vi "Forebrain - Final.vi"() -> ()   [LabVIEW 2012]
doc: "This VI contrains the Forebrain within the Olin Robot Architecture. It must be run first to load the appropriate mission definition files. It contains a finite state machine built around a tabbed Operator interface that will guide an operator through the startup, run shutdown mission sequence. After running it, run the Midbrain and Hindbrain VIS."
panel:
  in  "MapDarWithBuoys?":bool
  out "under cloud?":bool
  out "WhatAroundMeMap? Filtered":cluster{"T":dbl, "Range":dbl, "Bearing":dbl}[](array[cluster])
  out "Forebrain to Midbrain":T1
  in  "Upper Midbrain Active":bool
  out "Ir distance":i16
  in  "Midbrain Behavior weights":i8[](array[numeric])=[0, 0, 0, 0, 0, 0]
  in  "SOFT E-STOP":bool
  in  "Upper Midbrain Tweaks":T2={"Lider good scale mult"=0.00125, "Lider good scale add"=0.0, "Lider speed scale mult"=0.018, "Lider speed scale add"=0.0, "Follow right?"=FALSE, "IR Following Distance"=400, "IR scaling div"=50.0, "Lidar Cutoff"=0.0}
  out "Normalized Buoy Array":i32[][](array[numeric])
  in  "Buoy Array":i32[][](array[numeric])
  out "Number Waypoints":i32
  out "NXT String Sent":string="$B^"
  in  "Soft E-Stop":bool
  out "NXT String Received":string
  out "return count":u32
  out "error out":errorcluster
  in  "error in 2":errorcluster
  out "Desired \nVelocity":i16=5
  out "Ycurrent":dbl format="%#_3g"
  out "Xcurrent":dbl format="%#_3g"
  out "Ystart":dbl
  out "Xstart":dbl
  in  "error in":errorcluster
  out "Robot Live":bool
  in  "E-Stop":bool
  in  "Tab":T3(tab)
  out "MissionTime (Min)":dbl(knob) scale=0.0..10.0
  out "LidarDist":i16
  out "IR Index":i32
  out "BatteryLevel":dbl(slide) scale=6.0..9.0
  out "String Received":string
  out "Send String":string="$B^"
  in  "VISA resource name":refnum<visa-resource-name>="COM6"
  in  "Mode":i16 min=0 max=99 step=1
  in  "Desired Vel":i16(slide)=7 scale=0.0..14.0
  in  "Local Head":i16(slide)=7 scale=0.0..14.0
  out "StartMissionMap":picture
  out "MapDARCheck":picture
  in  "RunRobot":bool
  in  "Tug letter":string="G"
  out "Tug X":i32
  out "Tug Y":i32
  out "Tug H":i32
  out "BS Time Out?":bool
  out "Buoy locations":cluster{"regular expression":string, i32, i32}[](array[cluster])
  out "Valid ?":bool
  out "Battery\nVolts":i16
  out "Base Station data rec'd":string
  out "udp rate":bool
  out "CollisionWarning":bool
  out "DebugMapDAR":picture
  in  "MapDAR Control":T4={"NumberOfBeams"=180, "SensorRange"=500.0, "Noise (0.1 to 1)"=0.0} {"Noise (0.1 to 1)" min=0.0 max=1.0 step=0.1; "SensorRange" min=500.0 max=1500.0 step=100.0; "NumberOfBeams" min=36 max=360 step=2}
  out "MapDAR Data (r:pixel b:degrees)":cluster{"Range":dbl, "Bearing":dbl}[](array[cluster])
  in  "Stop DebugSENSE":bool
  out "MissionMap":picture
  out "Tug position":T5
  out "initialized MDF":T6(array[cluster])
  out "Way Point Index":i32
  out "InitialWaypoint":cluster{"X":i16, "Y":i16}
  in  "Pen Color":u32(colorbox)=15671808
  in  "Select Pen Attributes":T7={"Width"=1, "Style"=enum."Solid"}
  out "Draw??":bool
  in  "WhereAmI?FromBase":T8
  out "(xr,yr)":cluster{"X":dbl, "Y":dbl}
  in  "RobotPosition":T5 {"xrobot" min=0.0 max=1177.0 step=10.0; "yrobot" min=0.0 max=850.0 step=10.0; "heading" min=0.0 max=7.0 step=0.1}
  out "MDF_Original":T6(array[cluster])
  out "WhatAroundMeMap?":cluster{"T":dbl, "Range":dbl, "Bearing":dbl}[](array[cluster])
  out "WayPointAct":dbl[](array[numeric])
  out "SteerAngle":dbl
  out "MissionDefFile":picture
  out "MDF":T6(array[cluster])
  in  "Select Your Behavior":T9(ring)
  out "No. of Waypoints":i32
  in  "Exit Planning":bool
  in  "BoatSpeed for Leg":dbl(slide)=8.0 min=-9.0 max=9.0 step=1.0 scale=0.0..14.0
  out "BuildMDF":bool
  out "WayPoint Position":cluster{"X":i32, "Y":i32}
  out "Send String to NXT":string="$B^"
  in  "Behavior Command":T9(ring)
  out "CollisionLight":bool
  out "Where? Manual":T8
  out "ActManual":bool
  in  "Manual Heading":i16(knob)=7 min=0 max=14 step=1
  out "MWhat?":bool
  out "Where? 2":bool
  out "How? 2":bool
  in  "ManualModeStop":bool
  out "ManualModeMapDAR":picture
  out "ManualMissionMap":picture
  out "Battery":dbl(slide) scale=0.0..8.0
  in  "Manual Vel":dbl(slide)=7.0 min=0.0 max=14.0 step=1.0 scale=0.0..14.0
  out "MissionTime":dbl(knob) scale=0.0..10.0
  out "Heading":cluster{dbl, dbl}(knob)={0.0, 34.390870865624734} scale=180.0..-179.0 scale format="%#_3g"
  out "Speed":i16(knob) scale=-6.0..6.0
  out "Current Behavior":T9(ring)
  out "Robot Position":cluster{"X":dbl, "Y":dbl} {"X" format="%#_3g"; "Y" format="%#_3g"}
  out "Ready":bool
  in  "Pause":bool
  in  "Rerun MDF":bool
  out "CollisionLight 2":bool
  out "Act":bool
  out "Neo-C":bool
  out "How?":bool
  out "What?":bool
  out "A Heading":cluster{dbl, dbl}(knob)={0.0, 34.390870865624734} scale=180.0..-180.0
  out "A Speed":dbl(knob) scale=-9.0..9.0
  out "AutoBattery":dbl(slide) scale=0.0..8.0
  out "AutoModeLIDAR":picture
  out "AutoMissionMap":picture
  in  "RunAutoMode":bool
  out "MissionTimeAuto":dbl(knob) scale=0.0..60.0
  out "Where?":bool
  in  "WAYPOINT\n MODE":dbl=1.0
  in  "Current Waypoint":dbl
  in  "Manual\nOverride":bool=TRUE
  in  "Destinations Array":i64[][](array[numeric])=[[120, 280, 700, 408], [30, 140, 250, 400], [217, 811, 641, 816]]
  out "BAM Mission Map":picture
  out "Pixel X":dbl
  out "Pixel Y":dbl
  out "Direction":dbl
  out "Base Station String":string
  out "Battery Level":dbl
  in  "Heading":i16(knob)=7
  in  "Velocity":i16(slide)=7 scale=0.0..14.0
  out "Local\nHeading":i16=90
  # "To run\nrobot,\nclick\narrow\nabove\n\nRun Robot button must be on"
  # "Operation Directions\n\n1)Click on Startup&\nShutdown tab.\n2) Click on Run \nArrow on menubar.\nRun Forebrain,\nvis from the project\nexplorer.\n3) Select a mssion \nmap file when asked.\n4) Check robot is \nfully operational on\nStartup tab.\n5) Debug with debug\ntabs as required.\n6) Select ManualMode\ntab and test drive \nrobot.\n7) Select PlanMission\ntab and set up \nmission.\n8) Go to AutoMode\ntab and run mission."
  # "Turns off drive\nmotors"
  # "forebrain"
  # "wall follow"
  # "wall avoid"
  # "under cloud"
  # "GTFO"
  # "tend straight"
  # "inactive behaviors = 0\nstrongest behavior = 10"
  # "under cloud should always be zero"
  # "under cloud?"
  # "Enter Olin Test  Pool"
  # "Xbee Com Port"
  # "xBee\"Send String\" (mode, desired velocity, local heading)"
  # "(Type in Tug Letter  L T G P  (look at boat cradle)"
  # "Should be on to\nrun"
  # "BoatG,X,Y,H,BoatT,X,Y,H,BoatP,X,Y.H,BoatL,X,Y,H,BuoyA,X,Y,BuoyB,X,Y,BuoyC,X,Y,BuoyD,X,Y,Time(hours,Min,Sec)"
  # "To stop  program \nturn off here"
  # "Use this tab\nto explore\nLIDAR\ndata and \noperation"
  # "Set\nNumberOfBeams\nSensorRange\nNoise\nto\nview\nsimulated\nsensor\ndata"
  # "Turn Debug Sim \nto leave this\ntab--->"
  # "This tab will auto\nreturn to Startup \nin 2 seconds"
  # "Clean up interface and make more useful for debugging behaviors"
  # "Build out interface and make more useful for debugging act"
  # "This tab will auto\nreturn to Startup \nin 2 seconds"
  # "Directions:\n1) Select Robot Behavior for each mission leg.\n2) Select Robot Speed for leg.\n3) Click on robots current location for first waypoint.\n4) Hold down button and drag to next\nwaypoint. Click on next leg waypoint.\n5) Hold mouse button down and drag to \nnext waypoint. \n6) Click on next waypoint. Repeat for full mission.\n7) MDF will store up to 20 waypoints."
  # "Remember to\nset boat\nleg speed !"
  # "Please Adjust Scroll Barrs in Tug Off Mode to Prevent  Extra Lines Being Drawn"
  # "\"Send String\" (mode, desired velocity, local heading)"
  # "Press to stop and return to StartUp"
  # "Open MidBrain\nArbiter to see\nBrain Waves"
  # "AutoMode\nAutomatically \nReturns to \nStartUp Mode"
  # "Pixel coordinates for destinations."
  # "BoatG,X,Y,H,BoatT,X,Y,H,BoatP,X,Y.H,BoatL,X,Y,H,BuoyA,X,Y,BuoyB,X,Y,BuoyC,X,Y,BuoyD,X,Y,Time(hours,Min,Sec)"
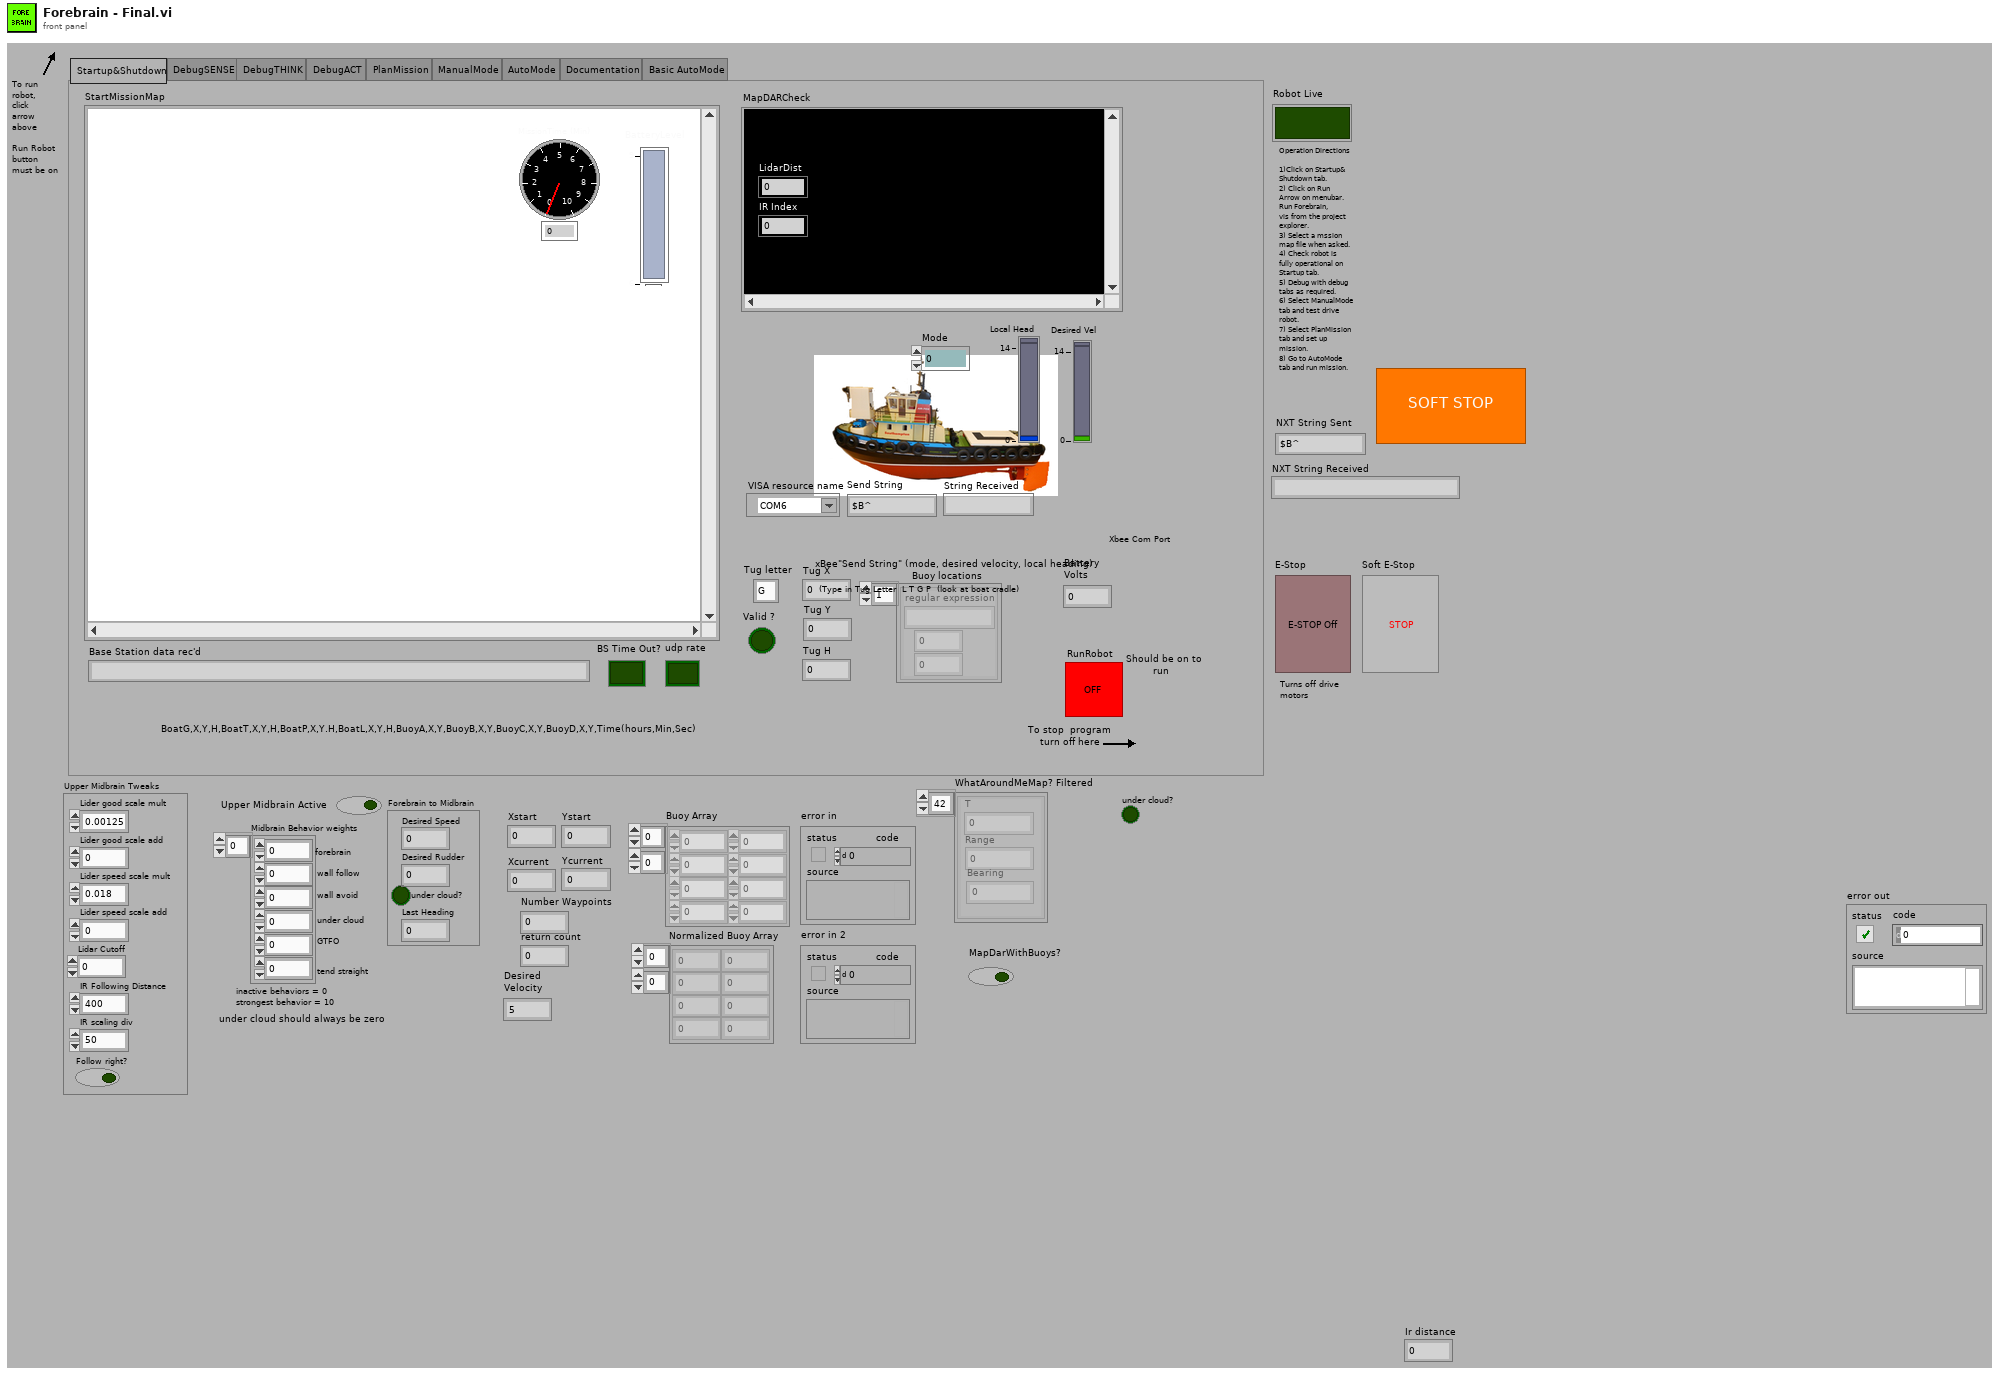
[diagram p1: front panel]
types:
  T1 = cluster{"Desired Speed":i16, "Desired Rudder":i16, bool, "Last Heading":i16}
  T2 = cluster{"Lider good scale mult":dbl, "Lider good scale add":dbl, "Lider speed scale mult":dbl, "Lider speed scale add":dbl, "Follow right?":bool, "IR Following Distance":i32, "IR scaling div":dbl, "Lidar Cutoff":dbl}
  T3 = enum32{"Startup&Shutdown", "DebugSENSE", "DebugTHINK", "DebugACT", "PlanMission", "ManualMode", "AutoMode", "Documentation", "Basic AutoMode"}
  T4 = cluster{"NumberOfBeams":i32, "SensorRange":dbl, "Noise (0.1 to 1)":dbl}
  T5 = cluster{"xrobot":dbl, "yrobot":dbl, "heading":dbl}
  T6 = cluster{"Status":enum16{"Past", "Current", "Future"}, "x":dbl, "y":dbl, "z":dbl, "Vel":dbl, "Dwell Time":dbl, "BehCom":enum16{"Tug Off", "Manual Mode", "Goto WayPoint", "Back Up", "Circle", "Left Wall Follow", "Right Wall Follow", "Hunt"}, "Expand1":dbl, "Expand2":dbl, "Expand3":dbl}[]
  T7 = cluster{"Width":u16, "Style":enum32{"Solid", "Dash", "Dot", "DashDot", "DashDotDot"}}
  T8 = cluster{"T":dbl, "X":dbl, "Y":dbl, "Direction":dbl}
  T9 = enum16{"Tug Off", "Manual Mode", "Goto WayPoint", "Back Up", "Circle", "Left Wall Follow", "Right Wall Follow", "Hunt"}
  T10 = enum32{"Startup&Shutdown", "DebugSENSE", "DebugTHINK", "DebugACT", "PlanMission", "ManualMode", "AutoMode", "Documentation"}
  T11 = cluster{"VelCom":dbl, "BehCom":enum16{"OpenFieldTransit", "P-WallFollow", "S-WallFollow", "LaneFollow", "ManualMode"}}
  T12 = typedef "IMAQ Image.ctl" = refnum<image>
  T13 = typedef "imagedata.ctl" = cluster{"image type":i32, "image depth":i32, "image":u8[], "mask":u8[], "colors":u32[], "Rectangle":cluster{"left":i16, "top":i16, "right":i16, "bottom":i16}}
  T14 = cluster{"Status":enum16{"Past", "Current", "Future"}, "x":dbl, "y":dbl, "z":dbl, "Vel":dbl, "Dwell Time":dbl, "BehCom":enum16{"Tug Off", "Manual Mode", "Goto WayPoint", "Back Up", "Circle", "Left Wall Follow", "Right Wall Follow", "Hunt"}, "Expand1":dbl, "Expand2":dbl, "Expand3":dbl}
  T15 = typedef "LVMouseTypeDef.ctl" = cluster{"Mouse Position":cluster{"X":i32, "Y":i32}, "Mouse Modifiers":cluster{"Button Down":bool, "Shift Mod":bool, "Menu Mod":bool, "Option Mod":bool}}
  T16 = cluster{"RudderAngle":i16, "t":i16, "under cloud?":bool, "Heading":i16}
  T17 = cluster{"regular expression":string, i32, i32, i32}
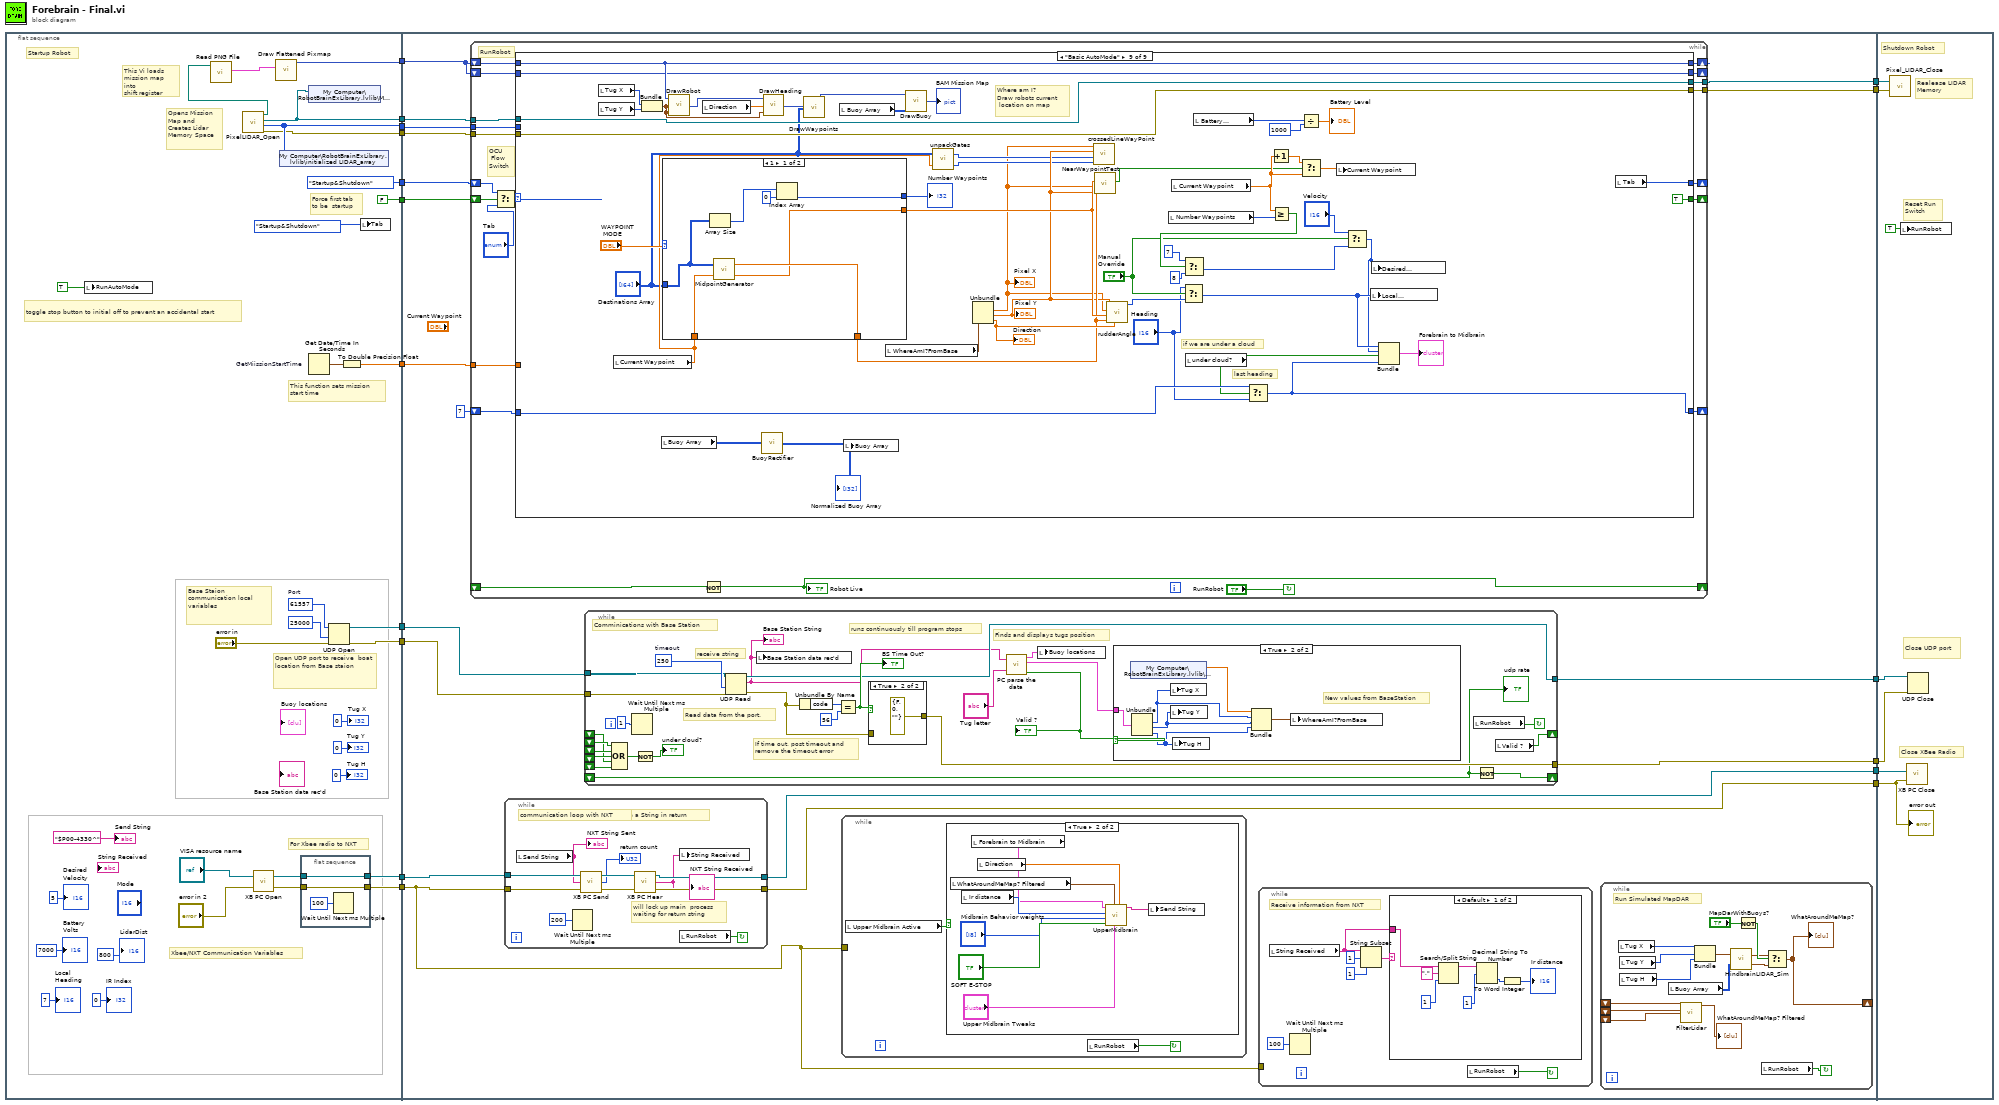
[diagram p0: block diagram]
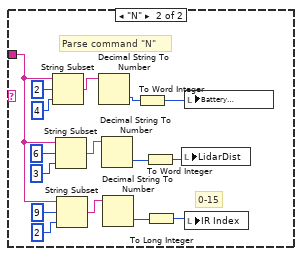
[diagram p2: hidden frame]
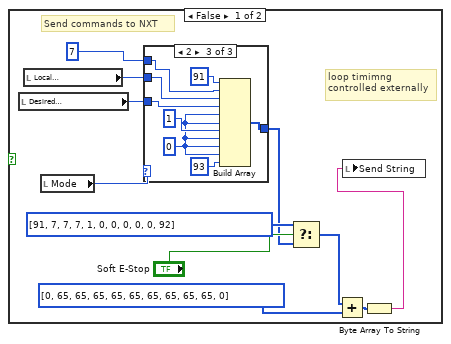
[diagram p3: hidden frame]
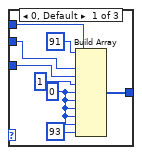
[diagram p4: hidden frame]
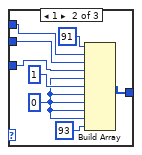
[diagram p5: hidden frame]
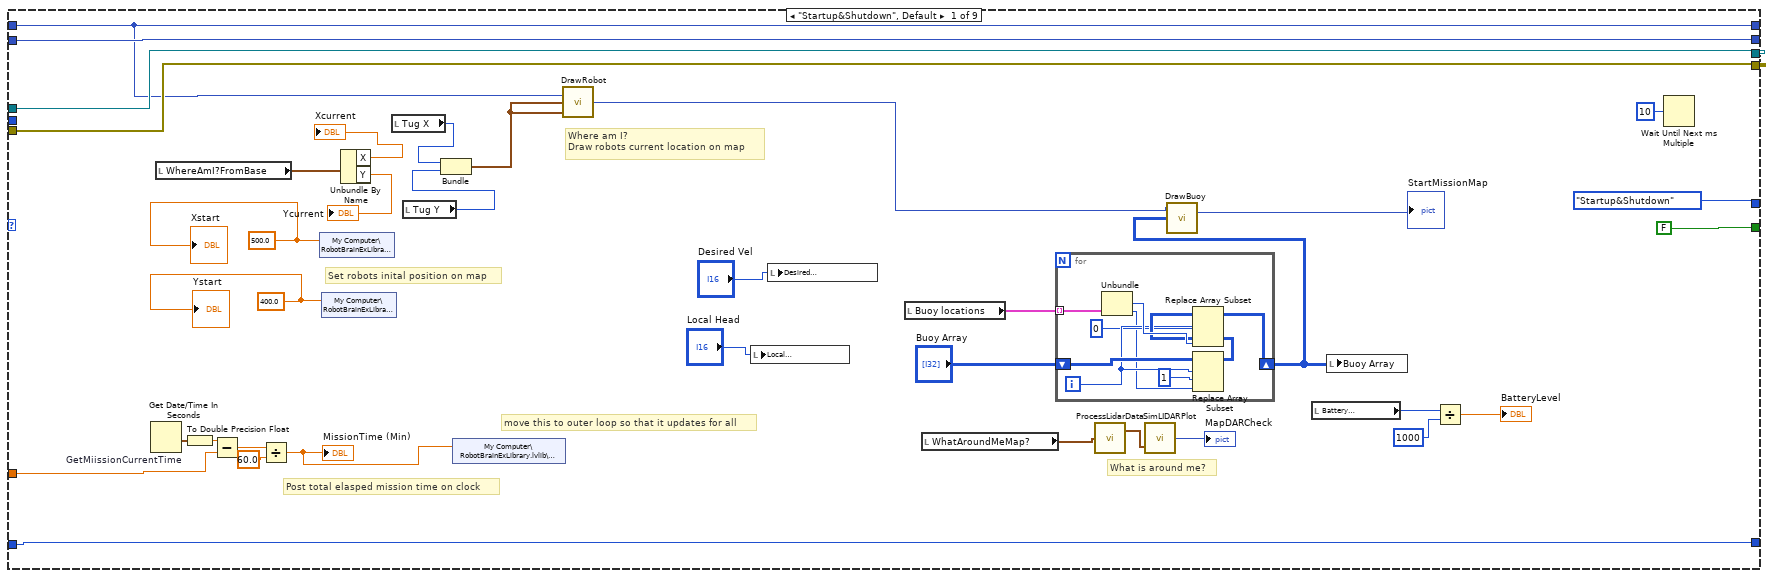
[diagram p8: hidden frame]
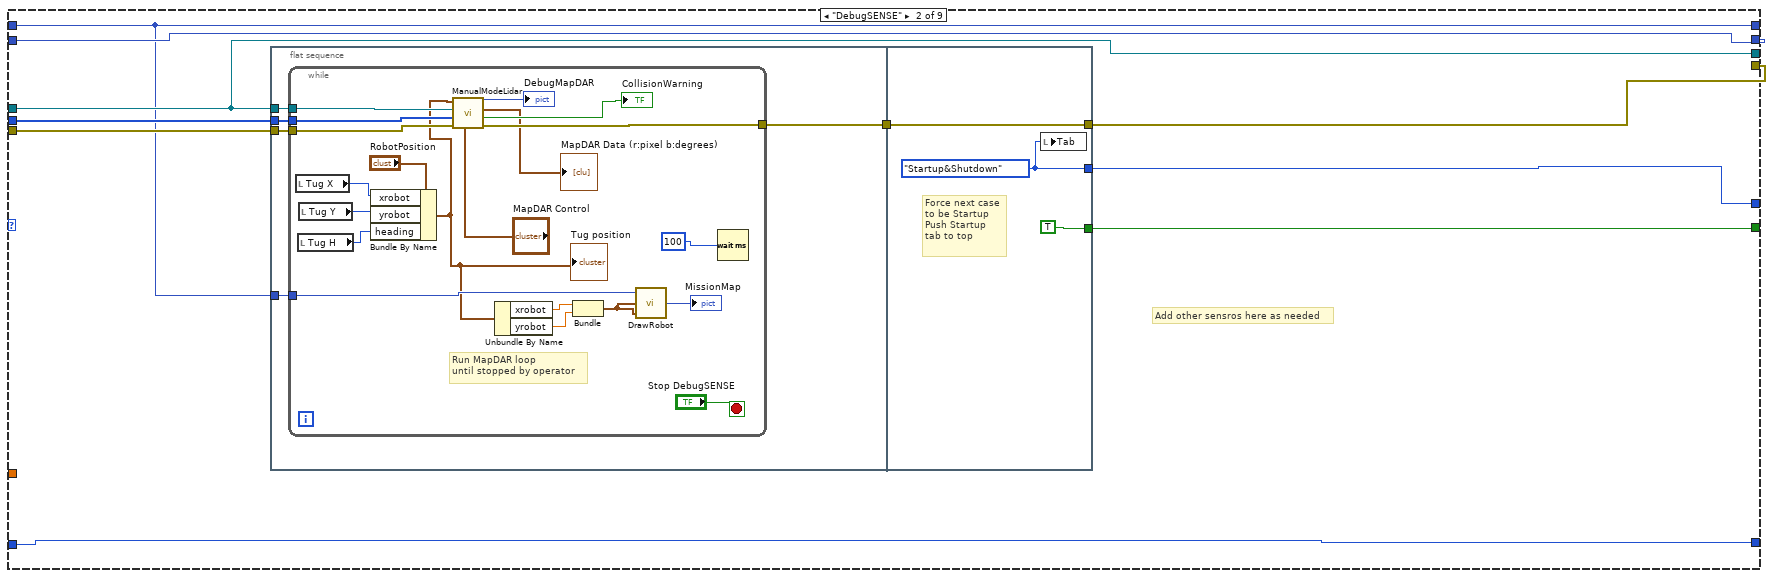
[diagram p9: hidden frame]
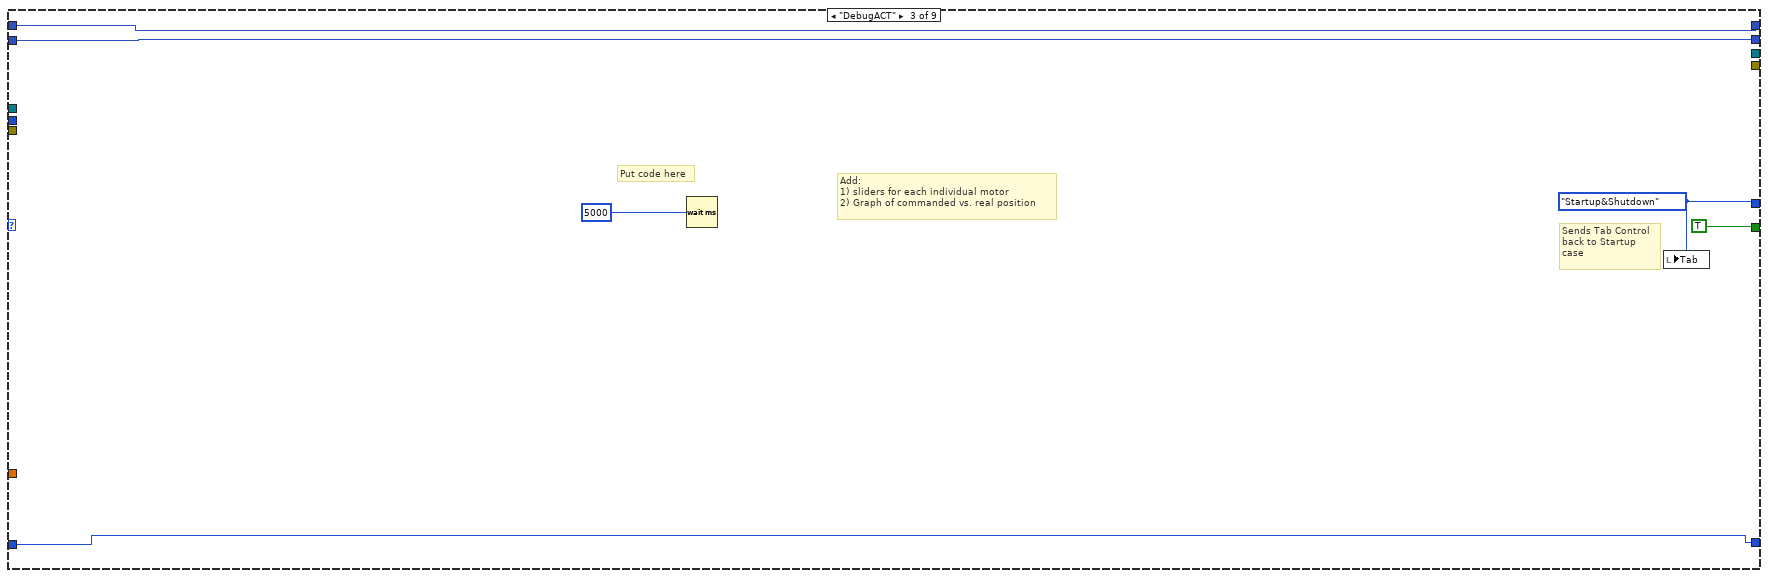
[diagram p10: hidden frame]
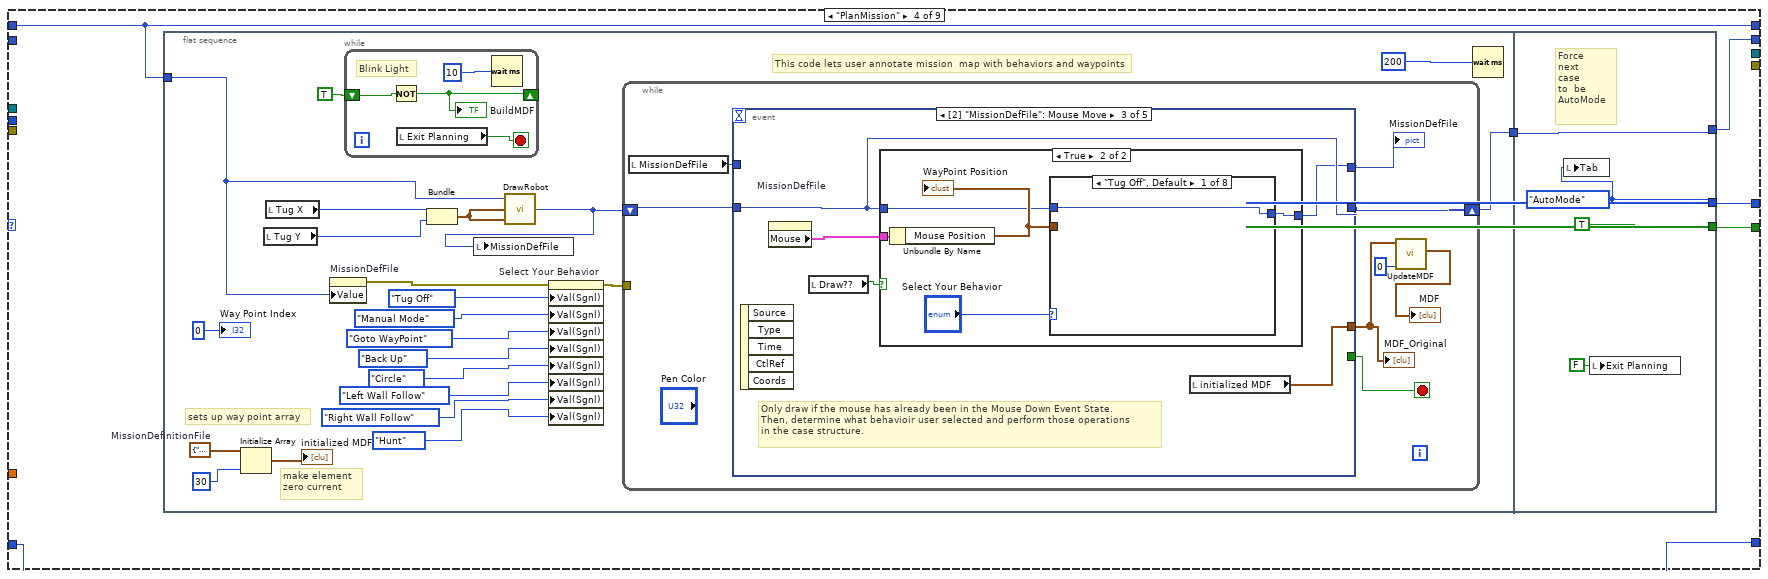
[diagram p11: hidden frame]
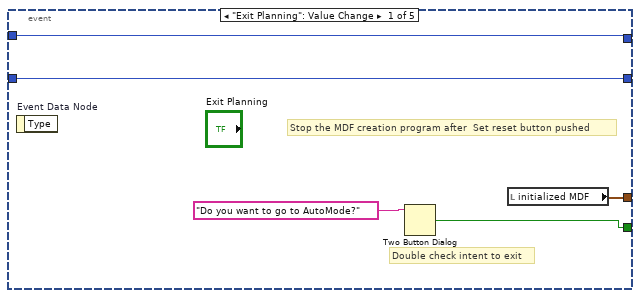
[diagram p12: hidden frame]
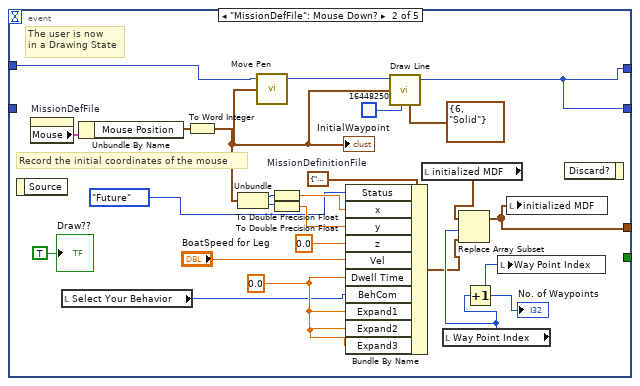
[diagram p13: hidden frame]
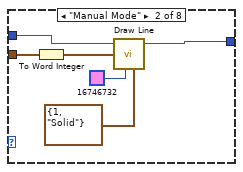
[diagram p15: hidden frame]
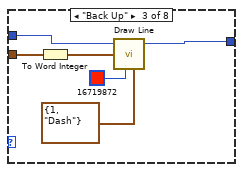
[diagram p16: hidden frame]
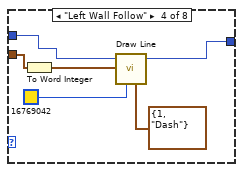
[diagram p17: hidden frame]
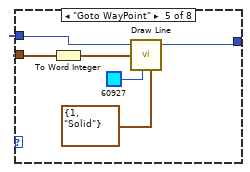
[diagram p18: hidden frame]
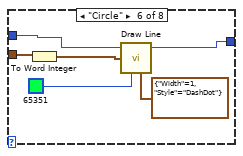
[diagram p19: hidden frame]
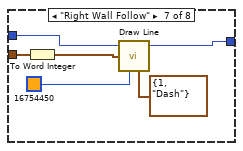
[diagram p20: hidden frame]
diagram:
  n1 = flat-sequence {
    tunnel: [w48] -> w17
    tunnel: [w47] -> w16
    tunnel: [w44] -> w15
    tunnel: [w46] -> w14
    tunnel: [w45] -> w13
    tunnel: [FALSE ("RunAutoMode")] -> w10
    tunnel: [T10."Startup&Shutdown" ("Tab")] -> w9
    tunnel: [w31] -> w8
    tunnel: [w30] -> w7
    tunnel: [w19] -> w6
    tunnel: [w18] -> w5
    tunnel: w17 -> [w70]
    tunnel: w16 -> [w69]
    tunnel: w15 -> [w68]
    tunnel: w14 -> [w67]
    tunnel: w13 -> [w66]
    tunnel: [w65] -> w12
    tunnel: [w64] -> w11
    tunnel: w10 -> [w63]
    tunnel: w9 -> [w62]
    tunnel: w8 -> [w57]
    tunnel: w7 -> [w56]
    tunnel: w6 -> [w61]
    tunnel: w5 -> [w58]
    tunnel: [w60] -> w4
    tunnel: [w59] -> w3
    tunnel: [w55] -> w2
    tunnel: [w54] -> w1
    tunnel: w12 -> [w738]
    tunnel: w11 -> [w737]
    tunnel: w4 -> [w736]
    tunnel: w3 -> [w735]
    tunnel: w2 -> [w734]
    tunnel: w1 -> [w733]
    frame #0 {
      w37 = u16 61557  # Port
      # "For Xbee radio to NXT"
      # "Xbee/NXT Communication Variables"
      # "Base Staion communication local variables"
      # "Open UDP port to receive  boat location from Base staion"
      # "Force first tab\nto be  startup"
      # "toggle stop button to initial off to prevent an accidental start"
      # "Opens Mission\nMap and\nCreates Lidar\nMemory Space"
      # "This function sets mission \nstart time"
      # "This Vi loads\nmission map into \nshift register"
      # "Startup Robot"
      n2 = local write "RunAutoMode"(TRUE ("RunAutoMode")) -> ()
      n3 = call "PixelLIDAR_Open.vi"() -> ("error out"=w45:errorcluster, "initialized LIDAR\narray"=w46:i32[], "MDF Image"=w44:T12, "MissionMap"=w39:path)  [unwired: 2 in]
      n4 = call <vilib>:"Read PNG File.vi"("path to PNG file"=w39) -> ("image data"=w38:T13)  [unwired: 8 in, 2 out]
      n5 = call "XB PC Open.vi"("error in (no error)"="error in 2", "VISA resource name"="VISA resource name") -> ("error out"=w22:errorcluster, "VISA resource name out"=w23:refnum<visa-resource-name>)
      n6 = call <vilib>:"Draw Flattened Pixmap.vi"("image data"=w38) -> ("new picture"=w47:picture)  [unwired: 8 in]
      n7 = shared-variable "My Computer\\RobotBrainExLibrary.lvlib\\initialized LIDAR_array"(w46) -> ()  [unwired: 1 in, 1 out]
      n8 = flat-sequence {
        tunnel: w23 -> [w50]
        tunnel: w22 -> [w51]
        tunnel: [w51] -> w18
        tunnel: [w50] -> w19
        frame #0 {
          n9 = Wait Until Next ms Multiple(millisecond multiple=u32 100) -> ()  [unwired: 1 out]
        }
      }
      n10 = shared-variable "My Computer\\RobotBrainExLibrary.lvlib\\MDF Image"(w44) -> ()  [unwired: 1 in, 1 out]
      n11 = Get Date/Time In Seconds "GetMiissionStartTime"() -> (seconds since 1Jan1904=w49:timestamp)
      n12 = UDP Open(8:"error in", 9:25000 ("timeout ms (25000)"), 11:w37) -> (port=w31:refnum<k16>, 0:w30:errorcluster)  [unwired: 2 in, 1 out]
      n13 = To Double Precision Float(number=w49) -> (double precision float=w48:dbl)
      n14 = local write "Tab"(T10."Startup&Shutdown" ("Tab")) -> ()
      "Tug X" <- 0 ("Tug X")
      "Tug Y" <- 0 ("Tug Y")
      "Tug H" <- 0 ("Tug H")
      "Battery\nVolts" <- i16 7000 ("Battery\nVolts")
      "LidarDist" <- i16 800 ("Dist")
      "IR Index" <- 0 ("IR Index")
      "Local\nHeading" <- i16 7 ("Local\nHeading")
      "Desired \nVelocity" <- i16 5 ("Desired \nVelocity")
      "Send String" <- "$P00-4330^"
    }
    frame #1 {
      n15 = while {
        shift-right: [w208] -> _
        shift-left: _ -> [w224]
        shift-right: [w223] -> _
        shift-left: w62 -> [w222]
        shift-right: [w219] -> _
        shift-left: w63 -> [w218]
        tunnel: w70 -> [w217]
        shift-right: [w207] -> _
        shift-left: w69 -> [w216]
        shift-right: [w214] -> _
        shift-left: w69 -> [w215]
        tunnel: w68 -> [w213]
        tunnel: w67 -> [w212]
        tunnel: w66 -> [w211]
        tunnel: [w210] -> w65
        tunnel: [w209] -> w64
        shift-right: [w206] -> _
        shift-left: i16 7 ("Heading") -> [w205]
        stop <- "RunRobot" continue-if-true
        # "RunRobot"
        # "OCU\n Flow\nSwitch"
        n16 = Select(t=w222, s=w218, f="Tab") -> (s? t:f=w220:T3)
        n17 = case shown="\"Basic AutoMode\"" w220 {
          selector: w220 -> [_ _ _ _ _ w563 _ _ _]
          tunnel: [T10."Startup&Shutdown" ("Tab") w275 w311 w319 w487 w564 T10."Startup&Shutdown" ("Tab") w662 w704] -> w223
          tunnel: [FALSE ("s") w274 TRUE ("s") w318 w488 w562 FALSE ("s") TRUE ("s") TRUE ("s")] -> w219
          tunnel: w217 -> [w254 _ _ _ w485 w560 _ _ _]
          tunnel: w216 -> [w232 w271 w310 w315 w483 w557 w654 w660 w710]
          tunnel: w215 -> [w253 w272 w309 _ w484 w559 w653 w659 w709]
          tunnel: [w253 w272 w309 w316 w484 w559 w653 w659 w709] -> w214
          tunnel: w213 -> [w252 w273 _ _ _ _ _ _ w705]
          tunnel: w212 -> [_ w279 _ _ _ _ _ _ _]
          tunnel: w211 -> [w251 w278 _ _ _ _ _ _ w702]
          tunnel: [w252 w273 _ _ _ _ _ _ w705] -> w210
          tunnel: [w251 w277 _ _ _ _ _ _ w702] -> w209
          tunnel: [w232 w271 w310 w315 w483 w557 w654 w660 w710] -> w207
          tunnel: [w226 w270 w308 w314 w482 w556 w652 w658 w672] -> w206
          tunnel: w205 -> [w226 w270 w308 w314 w482 w556 w652 w658 w674]
          frame "Startup&Shutdown", Default {
            w243 = 400.0 ("Ystart")
            w244 = 500.0 ("Xstart")
            # "move this to outer loop so that it updates for all"
            # "Where am I?\nDraw robots current location on map"
            # "Post total elasped mission time on clock"
            # "What is around me?"
            # "Set robots inital position on map"
            n18 = Get Date/Time In Seconds "GetMiissionCurrentTime"() -> (seconds since 1Jan1904=w258:timestamp)
            n19 = local read "WhereAmI?FromBase"() -> (w233:T8)
            n20 = To Double Precision Float(number=w258) -> (double precision float=w257:dbl)
            n21 = Subtract(x=w257, y=w254) -> (x-y=w256:dbl)
            n22 = Divide(x=w256, y=60.0) -> (x/y=w250:dbl)
            "MissionTime (Min)" <- w250
            n23 = shared-variable "My Computer\\RobotBrainExLibrary.lvlib\\Xstart"(w244) -> ()  [unwired: 1 in, 1 out]
            n24 = shared-variable "My Computer\\RobotBrainExLibrary.lvlib\\Ystart"(w243) -> ()  [unwired: 1 in, 1 out]
            n25 = Unbundle By Name(w233) -> ("X"=→"Xcurrent":dbl, "Y"=→"Ycurrent":dbl)
            n26 = local read "Tug X"() -> (w242:i32)
            n27 = local read "Tug Y"() -> (w241:i32)
            n28 = Bundle("Tug X"=w242, "Tug Y"=w241) -> (w247:cluster{"Tug X":i32, "Tug Y":i32})  [unwired: 1 in]
            n29 = shared-variable "My Computer\\RobotBrainExLibrary.lvlib\\MissionTime"(w250) -> ()  [unwired: 1 in, 1 out]
            n30 = call "DrawRobot.vi"("(xr,yr) old"=w247, "(xr,yr) new"=w247, "2D Picture"=w232) -> ("new picture"=w231:picture)
            n31 = local write "Local\nHeading"("Local Head") -> ()
            n32 = local write "Desired \nVelocity"("Desired Vel") -> ()
            n33 = local read "Buoy locations"() -> (w229:cluster{"regular expression":string, i32, i32}[])
            n34 = local read "WhatAroundMeMap?"() -> (w234:cluster{"T":dbl, "Range":dbl, "Bearing":dbl}[])
            n35 = for {
              tunnel: w229 -> [w269] mode=indexing
              shift-right: [w265] -> w227
              shift-left: "Buoy Array" -> [w268]
              i -> [w263]
              n36 = Unbundle(w269) -> (w267:i32, w261:i32)  [unwired: 1 out]
              n37 = Replace Array Subset(array=w268, new element=w261, index (row)=w263, index (col)=1 ("index")) -> (w266:i32[][])
              n38 = Replace Array Subset(array=w266, new element=w267, index (row)=w263, index (col)=0 ("index")) -> (w265:i32[][])
            }
            n39 = call "ProcessLidarData.vi"("WhatAroundMe?MM"=w234) -> ("data array [mag, phase (deg)]"=w248:cluster{"magnitude":dbl, "phase":dbl}[])  [unwired: 1 out]
            n40 = call "SimLIDARPlot.vi"("data array [mag, phase (deg)]"=w248) -> ("SONAR"=→"MapDARCheck":picture)  [unwired: 1 in]
            n41 = call "DrawBuoy.vi"("Array"=w227, "2D Picture"=w231) -> ("new picture"=→"StartMissionMap":picture)  [unwired: 1 in]
            n42 = local read "Battery\nVolts"() -> (w238:i16)
            n43 = local write "Buoy Array"(w227) -> ()
            n44 = Divide(x=w238, y=i16 1000) -> (x/y=→"BatteryLevel":dbl)
            n45 = Wait Until Next ms Multiple(millisecond multiple=u32 10) -> ()  [unwired: 1 out]
            "Xstart" <- w244
            "Ystart" <- w243
          }
          frame "DebugSENSE" {
            # "Add other sensros here as needed"
            n46 = flat-sequence {
              tunnel: w279 -> [w284]
              tunnel: w278 -> [w283]
              tunnel: w273 -> [w282]
              tunnel: [w281] -> w276
              tunnel: w271 -> [w280]
              tunnel: [w307] -> w277
              tunnel: w276 -> [w307]
              tunnel: [w306] -> w275
              tunnel: [TRUE ("s")] -> w274
              frame #0 {
                n47 = while {
                  tunnel: w284 -> [w304]
                  tunnel: w283 -> [w303]
                  tunnel: w282 -> [w302]
                  tunnel: [w301] -> w281
                  tunnel: w280 -> [w295]
                  stop <- "Stop DebugSENSE" stop-if-true
                  # "Run MapDAR loop\nuntil stopped by operator"
                  n48 = local read "Tug X"() -> (w289:i32)
                  n49 = local read "Tug H"() -> (w290:i32)
                  n50 = local read "Tug Y"() -> (w288:i32)
                  n51 = Bundle By Name(cluster="RobotPosition", "xrobot"=w289, "yrobot"=w288, "heading"=w290) -> (w286:T5)
                  "Tug position" <- w286
                  n52 = call "ManualModeLidar.vi"("LIDARControl"="MapDAR Control", "error in"=w303, "initialized \nsonar ray\narray"=w304, "MDF Image"=w302, "SubPosition"=w286) -> ("error out"=w301:errorcluster, "Collision\nWarning"=→"CollisionWarning":bool, "LIDAR Data (r:pixel b:degrees)"=→"MapDAR Data (r:pixel b:degrees)":cluster{"Range":dbl, "Bearing":dbl}[], "LIDAR"=→"DebugMapDAR":picture)  [unwired: 1 in]
                  n53 = Unbundle By Name(w286) -> ("xrobot"=w293:dbl, "yrobot"=w292:dbl)
                  n54 = Bundle("xrobot"=w293, "yrobot"=w292) -> (w285:cluster{"xrobot":dbl, "yrobot":dbl})  [unwired: 1 in]
                  n55 = call "DrawRobot.vi"("(xr,yr) old"=w285, "(xr,yr) new"=w285, "2D Picture"=w295) -> ("new picture"=→"MissionMap":picture)
                  n56 = Wait (ms)(milliseconds to wait=u32 100) -> ()  [unwired: 1 out]
                }
              }
              frame #1 {
                w306 = T10."Startup&Shutdown" ("Tab")
                # "Force next case\nto be Startup\nPush Startup\ntab to top"
                n57 = local write "Tab"(w306) -> ()
              }
            }
          }
          frame "DebugACT" {
            w311 = T10."Startup&Shutdown" ("Tab")
            # "Add:\n1) sliders for each individual motor\n2) Graph of commanded vs. real position"
            # "Put code here"
            # "Sends Tab Control\nback to Startup\ncase"
            n58 = Wait (ms)(milliseconds to wait=u32 5000) -> ()  [unwired: 1 out]
            n59 = local write "Tab"(w311) -> ()
          }
          frame "PlanMission" {
            n60 = flat-sequence {
              tunnel: [w340] -> w317
              tunnel: w315 -> [w333]
              tunnel: [w480] -> w319
              tunnel: [TRUE ("s")] -> w318
              tunnel: w317 -> [w479]
              tunnel: [w479] -> w316
              frame #0 {
                w331 = T14 {"Status"=enum."Future", "x"=0.0, "y"=0.0, "z"=0.0, "Vel"=0.0, "Dwell Time"=0.0, "BehCom"=enum."Tug Off", "Expand1"=0.0, "Expand2"=0.0, "Expand3"=0.0}  # MissionDefinitionFile
                # "make element \nzero current"
                # "sets up way point array"
                # "This code lets user annotate mission  map with behaviors and waypoints"
                n61 = Initialize Array ("Initialize WaypointArray")(w331, 30 ("dimension size")) -> (→"initialized MDF":T6)
                n62 = local read "Tug Y"() -> (w328:i32)
                n63 = local read "Tug X"() -> (w329:i32)
                n64 = property on="MissionDefFile" class="Pict"("Value"=w333) -> (error out=w338:errorcluster)  [unwired: 2 in, 1 out]
                n65 = while {
                  shift-right: [w344] -> _
                  shift-left: TRUE -> [w345]
                  stop <- w343 stop-if-true
                  # "Blink Light"
                  n66 = Not(x=w345) -> (.not. x?=w344:bool)
                  "BuildMDF" <- w344
                  n67 = local read "Exit Planning"() -> (w343:bool)
                  n68 = Wait (ms)(milliseconds to wait=u32 10) -> ()  [unwired: 1 out]
                }
                n69 = Bundle("Tug X"=w329, "Tug Y"=w328) -> (w334:cluster{"Tug X":i32, "Tug Y":i32})  [unwired: 1 in]
                n70 = call "DrawRobot.vi"("(xr,yr) old"=w334, "(xr,yr) new"=w334, "2D Picture"=w333) -> ("new picture"=w332:picture)
                n71 = local write "MissionDefFile"(w332) -> ()
                n72 = property on="Select Your Behavior" class="Enum (strict)"(error in=w338, "Val(Sgnl)"=T9."Tug Off" ("Value (Signaling)"), "Val(Sgnl)"=T9."Manual Mode" ("Value (Signaling)"), "Val(Sgnl)"=T9."Goto WayPoint" ("Value (Signaling)"), "Val(Sgnl)"=T9."Back Up" ("Value (Signaling)"), "Val(Sgnl)"=T9."Circle" ("Value (Signaling)"), "Val(Sgnl)"=T9."Left Wall Follow" ("Value (Signaling)"), "Val(Sgnl)"=T9."Right Wall Follow" ("Value (Signaling)"), "Val(Sgnl)"=T9."Hunt" ("Value (Signaling)")) -> (error out=w339:errorcluster)  [unwired: 1 in, 1 out]
                n73 = while {
                  shift-right: [w352] -> w340
                  shift-left: w332 -> [w353]
                  tunnel: w339 -> [_]
                  stop <- w351 stop-if-true
                  n74 = local read "MissionDefFile"() -> (w350:picture)
                  n75 = event shown="[2] \"MissionDefFile\": Mouse Move" {
                    selector: _ -> [_ _ _ _ _]
                    dyn-events: _ -> [_ _ _ _ _]
                    timeout: _ -> [_ _ _ _ _]
                    tunnel: [w356 w364 w384 w437 w475] -> w352
                    tunnel: w353 -> [w356 _ w384 w437 _]
                    tunnel: [w357 _ _ _ _] -> w351
                    tunnel: [w355 w379 w385 w439 w476] -> w347
                    tunnel: w350 -> [w354 w365 _ w438 w475]
                    tunnel: [w354 w364 w383 w438 w475] -> w349
                    event "Exit Planning": Value Change {
                      # "Double check intent to exit"
                      # "Stop the MDF creation program after  Set reset button pushed"
                      n76 = event-data "Event Data Node"() -> ()  [unwired: 1 in, 1 out]
                      n77 = Two Button Dialog(message="Do you want to go to AutoMode?") -> (T button?=w357:bool)  [unwired: 2 in]
                      n78 = local read "initialized MDF"() -> (w355:T6)
                    }
                    event "MissionDefFile": Mouse Down? {
                      w363 = T14 {"Status"=enum."Future", "x"=0.0, "y"=0.0, "z"=0.0, "Vel"=0.0, "Dwell Time"=0.0, "BehCom"=enum."Tug Off", "Expand1"=0.0, "Expand2"=0.0, "Expand3"=0.0}  # MissionDefinitionFile
                      w373 = 0.0 ("Dwell Time")
                      # "Record the initial coordinates of the mouse"
                      # "The user is now\nin a Drawing State"
                      n79 = event-data() -> ()  [unwired: 1 in, 1 out]
                      n80 = property on="MissionDefFile" class="Pict"() -> ("Mouse"=w382:T15)  [unwired: 2 in, 2 out]
                      n81 = local read "Select Your Behavior"() -> (w360:T9)
                      n82 = Unbundle By Name(w382) -> ("Mouse Position"=w380:cluster{"X":i32, "Y":i32})
                      n83 = To Word Integer(number=w380) -> (16bit integer=w368:cluster{"X":i16, "Y":i16})
                      "InitialWaypoint" <- w368
                      n84 = Unbundle(w368) -> ("X"=w377:i16, "Y"=w376:i16)
                      n85 = call <vilib>:"Move Pen.vi"("new position"=w368, "picture"=w365) -> ("new picture"=w369:picture)  [unwired: 3 in]
                      n86 = To Double Precision Float(number=w377) -> (double precision float=w375:dbl)
                      n87 = To Double Precision Float(number=w376) -> (double precision float=w374:dbl)
                      n88 = Bundle By Name(cluster=w363, "Status"=enum16{"Past", "Current", "Future"}."Future", "x"=w375, "y"=w374, "z"=0.0, "Vel"="BoatSpeed for Leg", "Dwell Time"=w373, "BehCom"=w360, "Expand1"=w373, "Expand2"=w373, "Expand3"=w373) -> (w359:T14)
                      n89 = call <vilib>:"Draw Line.vi"("picture"=w369, "end point"=w368, "color(black)"=u32 16448250, "pen"=T7 {"Width"=6, "Style"=enum."Solid"}) -> ("new picture"=w364:picture)  [unwired: 5 in]
                      n90 = local read "initialized MDF"() -> (w378:T6)
                      n91 = local read "Way Point Index"() -> (w361:i32)
                      n92 = Replace Array Subset(array=w378, new element=w359, index=w361) -> (w379:T6)
                      n93 = Increment(x=w361) -> (x+1=w381:i32)
                      "No. of Waypoints" <- w381
                      n94 = local write "Way Point Index"(w381) -> ()
                      n95 = local write "initialized MDF"(w379) -> ()
                      n96 = event-data() -> ()  [unwired: 2 in, 1 out]
                      "Draw??" <- TRUE ("Draw??")
                    }
                    event "MissionDefFile": Mouse Move {
                      # "Only draw if the mouse has already been in the Mouse Down Event State.\nThen, determine what behavioir user selected and perform those operations\nin the case structure."
                      n97 = event-data() -> ()  [unwired: 1 in, 5 out]
                      n98 = property on="MissionDefFile" class="Pict"() -> ("Mouse"=w387:T15)  [unwired: 2 in, 2 out]
                      n99 = local read "Draw??"() -> (w386:bool)
                      n100 = case shown="True" w386 {
                        tunnel: w387 -> [_ w393]
                        tunnel: w384 -> [w388 w389]
                        tunnel: [w388 w390] -> w383
                        frame False {
                        }
                        frame True {
                          n101 = Unbundle By Name(w393) -> ("Mouse Position"=w391:cluster{"X":i32, "Y":i32})
                          "WayPoint Position" <- w391
                          n102 = case shown="\"Tug Off\", Default" "Select Your Behavior" {
                            tunnel: w391 -> [_ w399 w405 w408 w414 w419 w425 w431]
                            tunnel: [w394 w400 w406 w410 w413 w420 w426 w432] -> w390
                            tunnel: w389 -> [w394 w398 w402 w411 w415 w421 w427 w433]
                            frame "Tug Off", Default {
                            }
                            frame "Manual Mode" {
                              n103 = To Word Integer(number=w399) -> (16bit integer=w395:cluster{"X":i16, "Y":i16})
                              n104 = call <vilib>:"Draw Line.vi"("picture"=w398, "end point"=w395, "color(black)"=u32 16746732, "pen"=T7 {"Width"=1, "Style"=enum."Solid"}) -> ("new picture"=w400:picture)  [unwired: 5 in]
                            }
                            frame "Back Up" {
                              n105 = To Word Integer(number=w405) -> (16bit integer=w401:cluster{"X":i16, "Y":i16})
                              n106 = call <vilib>:"Draw Line.vi"("picture"=w402, "end point"=w401, "color(black)"=u32 16719872, "pen"=T7 {"Width"=1, "Style"=enum."Dash"}) -> ("new picture"=w406:picture)  [unwired: 5 in]
                            }
                            frame "Left Wall Follow" {
                              n107 = To Word Integer(number=w408) -> (16bit integer=w409:cluster{"X":i16, "Y":i16})
                              n108 = call <vilib>:"Draw Line.vi"("picture"=w411, "end point"=w409, "color(black)"=u32 16769042, "pen"=T7 {"Width"=1, "Style"=enum."Dash"}) -> ("new picture"=w410:picture)  [unwired: 5 in]
                            }
                            frame "Goto WayPoint" {
                              n109 = To Word Integer(number=w414) -> (16bit integer=w416:cluster{"X":i16, "Y":i16})
                              n110 = call <vilib>:"Draw Line.vi"("picture"=w415, "end point"=w416, "color(black)"=u32 60927, "pen"=T7 {"Width"=1, "Style"=enum."Solid"}) -> ("new picture"=w413:picture)  [unwired: 5 in]
                            }
                            frame "Circle" {
                              n111 = To Word Integer(number=w419) -> (16bit integer=w424:cluster{"X":i16, "Y":i16})
                              n112 = call <vilib>:"Draw Line.vi"("picture"=w421, "end point"=w424, "color(black)"=u32 65351, "pen"=T7 {"Width"=1, "Style"=enum."DashDot"}) -> ("new picture"=w420:picture)  [unwired: 5 in]
                            }
                            frame "Right Wall Follow" {
                              n113 = To Word Integer(number=w425) -> (16bit integer=w430:cluster{"X":i16, "Y":i16})
                              n114 = call <vilib>:"Draw Line.vi"("picture"=w427, "end point"=w430, "color(black)"=u32 16754450, "pen"=T7 {"Width"=1, "Style"=enum."Dash"}) -> ("new picture"=w426:picture)  [unwired: 5 in]
                            }
                            frame "Hunt" {
                              n115 = To Word Integer(number=w431) -> (16bit integer=w434:cluster{"X":i16, "Y":i16})
                              n116 = call <vilib>:"Draw Line.vi"("picture"=w433, "end point"=w434, "color(black)"=u32 16720896, "pen"=T7 {"Width"=1, "Style"=enum."DashDotDot"}) -> ("new picture"=w432:picture)  [unwired: 5 in]
                            }
                          }
                        }
                      }
                      n117 = local read "initialized MDF"() -> (w385:T6)
                    }
                    event "Select Your Behavior": Value Change {
                      # "When the user selects a new operation, we disable certain controls that aren't relevant to\nthe operation that the user is performing."
                      n118 = event-data() -> ("NewVal"=w442:T9)  [unwired: 1 in]
                      n119 = property on="Select Pen Attributes" class="Clust (strict)"() -> ("Controls[]"=w441:refnum<vi>[])  [unwired: 2 in, 2 out]
                      n120 = case shown="\"Manual Mode\"" w442 {
                        tunnel: w441 -> [w446 w447 w451 w455 w459 w463 w467 w471]
                        tunnel: "Select Pen Attributes" -> [_ _ _ _ _ _ _ _]
                        frame "Manual Mode" {
                          # "All attributes are valid for this\noperation."
                          n121 = Index Array "Index Array"(array=w446, index=1) -> (element=w444:refnum<vi>)
                          n122 = property on="Property Node" class="Ctl"(reference=w444, "Disabled"=u8 0) -> ()  [unwired: 1 in, 2 out]
                        }
                        frame "Back Up" {
                          # "All attributes are valid for this\noperation."
                          n123 = Index Array(array=w447, index=1) -> (element=w449:refnum<vi>)
                          n124 = property class="Ctl"(reference=w449, "Disabled"=u8 0) -> ()  [unwired: 1 in, 2 out]
                        }
                        frame "Tug Off" {
                          # "All attributes are valid for this\noperation."
                          n125 = Index Array "Index Array"(array=w451, index=1) -> (element=w453:refnum<vi>)
                          n126 = property on="Property Node" class="Ctl"(reference=w453, "Disabled"=u8 0) -> ()  [unwired: 1 in, 2 out]
                        }
                        frame "Left Wall Follow" {
                          # "All attributes are valid for this\noperation."
                          n127 = Index Array "Index Array"(array=w455, index=1) -> (element=w457:refnum<vi>)
                          n128 = property on="Property Node" class="Ctl"(reference=w457, "Disabled"=u8 0) -> ()  [unwired: 1 in, 2 out]
                        }
                        frame "Goto WayPoint" {
                          # "All attributes are valid for this\noperation."
                          n129 = Index Array "Index Array"(array=w459, index=1) -> (element=w461:refnum<vi>)
                          n130 = property on="Property Node" class="Ctl"(reference=w461, "Disabled"=u8 0) -> ()  [unwired: 1 in, 2 out]
                        }
                        frame "Circle" {
                          # "All attributes are valid for this\noperation."
                          n131 = Index Array "Index Array"(array=w463, index=1) -> (element=w465:refnum<vi>)
                          n132 = property on="Property Node" class="Ctl"(reference=w465, "Disabled"=u8 0) -> ()  [unwired: 1 in, 2 out]
                        }
                        frame "Right Wall Follow" {
                          # "All attributes are valid for this\noperation."
                          n133 = Index Array "Index Array"(array=w467, index=1) -> (element=w469:refnum<vi>)
                          n134 = property on="Property Node" class="Ctl"(reference=w469, "Disabled"=u8 0) -> ()  [unwired: 1 in, 2 out]
                        }
                        frame "Hunt" {
                          # "All attributes are valid for this\noperation."
                          n135 = Index Array "Index Array"(array=w471, index=1) -> (element=w473:refnum<vi>)
                          n136 = property on="Property Node" class="Ctl"(reference=w473, "Disabled"=u8 0) -> ()  [unwired: 1 in, 2 out]
                        }
                      }
                      n137 = local read "initialized MDF"() -> (w439:T6)
                    }
                    event "MissionDefFile": Mouse Up {
                      # "When the user is finished drawing, we complete the operation."
                      # "Finished Drawing"
                      n138 = event-data() -> ()  [unwired: 1 in, 3 out]
                      n139 = local write "Draw??"(FALSE ("Draw??")) -> ()
                      n140 = local read "initialized MDF"() -> (w476:T6)
                    }
                  }
                  "MissionDefFile" <- w349
                  "MDF_Original" <- w347
                  n141 = call "UpdateMDF.vi"("Index"=0, "MDF_In"=w347) -> ("MDF_Out"=→"MDF":T6)  [unwired: 9 in]
                }
                n142 = Wait (ms)(milliseconds to wait=u32 200) -> ()  [unwired: 1 out]
                "Way Point Index" <- 0 ("Boundary Point Index")
              }
              frame #1 {
                w480 = T10."AutoMode" ("Tab")
                # "Force \nnext \ncase\nto  be\nAutoMode"
                n143 = local write "Tab"(w480) -> ()
                n144 = local write "Exit Planning"(FALSE ("Exit Planning")) -> ()
              }
            }
          }
          frame "ManualMode" {
            # "Removing map shift register\nfixed memory leak?"
            # "Manual Steering by dashboard heading steering wheel\nand by speed slider"
            # "This mode lets \noperator directly\ndrive robot via\nthe ManualMode\ntabbed interface"
            n145 = while {
              shift-right: [w511] -> _
              shift-left: _ -> [w510]
              tunnel: w485 -> [w503]
              shift-right: [w500] -> _
              shift-left: _ -> [w499]
              tunnel: w483 -> [w497]
              stop <- w509 stop-if-true
              # "WhereAmI?"
              n146 = Get Date/Time In Seconds "GetMiissionCurrentTime"() -> (seconds since 1Jan1904=w504:timestamp)
              n147 = call "WhereForebrainPerception.vi"("Where? Midbrain"="WhereAmI?FromBase") -> ("Where? Forebrain"=→"Where? Manual":T8, "(xr,yr)"=w500:cluster{"X":dbl, "Y":dbl}, "Direction"=w489:dbl)  [unwired: 3 in, 1 out]
              "(xr,yr)" <- w500
              n148 = local read "ManualModeStop"() -> (w509:bool)
              n149 = To Double Precision Float(number=w504) -> (double precision float=w505:dbl)
              n150 = Greater Or Equal?(x=w489, y=181.0) -> (x >= y?=w494:bool)
              n151 = local read "Manual Heading"() -> (w501:i16)
              n152 = Subtract(x=w505, y=w503) -> (x-y=w506:dbl)
              n153 = Not(x=w510) -> (.not. x?=w511:bool)
              n154 = call "DrawRobot.vi"("(xr,yr) old"=w499, "(xr,yr) new"=w500, "2D Picture"=w497) -> ("new picture"=→"ManualMissionMap":picture)
              n155 = Divide(x=w506, y=60.0) -> (x/y=w508:dbl)
              "MissionTime" <- w508
              n156 = Subtract(x=w489, y=360.0) -> (x-y=w492:dbl)
              n157 = shared-variable "My Computer\\RobotBrainExLibrary.lvlib\\MissionTime"(w508) -> ()  [unwired: 1 in, 1 out]
              n158 = Select(t=w492, s=w494, f=w489) -> (s? t:f=w491:dbl)
              n159 = Bundle("Direction"=w491, "Manual Heading"=w501) -> (→"Heading":cluster{"Direction":dbl, "Manual Heading":i16})  [unwired: 1 in]
              n160 = Wait Until Next ms Multiple(millisecond multiple=u32 100 ("milliseconds to wait")) -> ()  [unwired: 1 out]
              "Where? 2" <- w510
            }
            n161 = while {
              shift-right: [w518] -> _
              shift-left: _ -> [w519]
              stop <- "ManualModeStop" stop-if-true
              # "WhatIsAroundMe?"
              n162 = local read "WhatAroundMeMap?"() -> (w513:cluster{"T":dbl, "Range":dbl, "Bearing":dbl}[])
              n163 = call "ProcessLidarData.vi"("WhatAroundMe?MM"=w513) -> ("Collision"=w514:bool, "data array [mag, phase (deg)]"=w515:cluster{"magnitude":dbl, "phase":dbl}[])
              "CollisionLight" <- w514
              n164 = Not(x=w519) -> (.not. x?=w518:bool)
              "MWhat?" <- w518
              n165 = call "SimLIDARPlot.vi"("data array [mag, phase (deg)]"=w515) -> ("SONAR"=→"ManualModeMapDAR":picture)  [unwired: 1 in]
              n166 = case shown="True" w514 {
                frame False {
                  # "No \nBeep"
                }
                frame True {
                  n167 = call <vilib>:"Beep.vi"("use system alert? (T)"=TRUE, "duration (msec)"=u32 1000, "frequency (Hz)"=u32 900) -> ()  [unwired: 9 in]
                }
              }
              n168 = Wait Until Next ms Multiple(millisecond multiple=u32 100 ("milliseconds to wait")) -> ()  [unwired: 1 out]
            }
            n169 = while {
              shift-right: [w543] -> _
              shift-left: _ -> [w542]
              stop <- w541 stop-if-true
              # "HowAmI?"
              n170 = local read "Battery\nVolts"() -> (w540:i16)
              n171 = local read "ManualModeStop"() -> (w541:bool)
              n172 = Not(x=w542) -> (.not. x?=w543:bool)
              n173 = Divide(x=w540, y=i16 1000) -> (x/y=→"Battery":dbl)
              n174 = Wait Until Next ms Multiple(millisecond multiple=u32 100 ("milliseconds to wait")) -> ()  [unwired: 1 out]
              "How? 2" <- w542
            }
            n175 = while {
              shift-right: [w537] -> _
              shift-left: _ -> [w536]
              stop <- w535 stop-if-true
              # "ForebrainAct"
              n176 = local read "E-Stop"() -> (w533:bool)
              n177 = local read "ManualModeStop"() -> (w535:bool)
              n178 = Select(t=0.0, s=w533, f="Manual Vel") -> (s? t:f=w530:dbl)
              n179 = To Word Integer(number=w530) -> (16bit integer=w528:i16)
              "Speed" <- w528
              n180 = local read "Send String"() -> (→"Send String to NXT":string)
              n181 = To Word Integer(number="Behavior Command") -> (16bit integer=w525:i16)
              n182 = local write "Upper Midbrain Active"("Upper Midbrain Active") -> ()
              n183 = local write "Mode"(w525) -> ()
              n184 = local write "Desired \nVelocity"(w528) -> ()
              n185 = local write "Local\nHeading"("Manual Heading") -> ()
              n186 = Not(x=w536) -> (.not. x?=w537:bool)
              n187 = Wait Until Next ms Multiple(millisecond multiple=u32 50 ("milliseconds to wait")) -> ()  [unwired: 1 out]
              "ActManual" <- w536
            }
            n188 = local read "ManualModeStop"() -> (w486:bool)
            n189 = case shown="True" w486 {
              tunnel: [TRUE ("s") w547] -> w488
              tunnel: [T10."ManualMode" ("Tab") w548] -> w487
              frame False {
              }
              frame True {
                # "Debounce tab for clean transition"
                n190 = flat-sequence {
                  tunnel: [w554] -> w548
                  tunnel: [TRUE ("s")] -> w547
                  frame #0 {
                    n191 = Wait (ms)(milliseconds to wait=u32 100) -> ()  [unwired: 1 out]
                  }
                  frame #1 {
                    w554 = T10."Startup&Shutdown" ("Tab")
                    # "Turn off\nVelocity\non \nExit"
                    n192 = local write "ManualModeStop"(FALSE ("ManualModeStop")) -> ()
                    n193 = local write "Desired \nVelocity"(i16 0 ("Desired \nVelocity")) -> ()
                    n194 = local write "Local\nHeading"(i16 0 ("Local\nHeading")) -> ()
                    n195 = local write "Mode"(i16 0 ("Mode")) -> ()
                    n196 = local write "Tab"(w554) -> ()
                  }
                }
              }
            }
          }
          frame "AutoMode" {
            n197 = flat-sequence {
              tunnel: w563 -> [_]
              tunnel: [w566] -> w561
              tunnel: w560 -> [w566]
              tunnel: w559 -> [w565]
              tunnel: [w565] -> w558
              tunnel: w557 -> [_]
              tunnel: w561 -> [w573]
              tunnel: w558 -> [w571]
              tunnel: [w650] -> w564
              tunnel: [FALSE ("s")] -> w562
              frame #0 {
                # "Run Robot\nbased on\nmission\ndefinition\nfile"
                n198 = local write "AutoMissionMap"(w565) -> ()
                n199 = while {
                  shift-right: [w569] -> _
                  shift-left: _ -> [w568]
                  stop <- "RunAutoMode" continue-if-true
                  # "Wait for Run\nbutton press\nbefore\nturning on\nAutoMode\nCode"
                  n200 = Not(x=w568) -> (.not. x?=w569:bool)
                  n201 = Wait Until Next ms Multiple(millisecond multiple=u32 100 ("milliseconds to wait")) -> ()  [unwired: 1 out]
                  "Ready" <- w568
                }
              }
              frame #1 {
                n202 = while {
                  shift-right: [w619] -> _
                  shift-left: _ -> [w610]
                  tunnel: w573 -> [w614]
                  shift-right: [w612] -> _
                  shift-left: _ -> [w613]
                  tunnel: w571 -> [w605]
                  stop <- w609 stop-if-true
                  # "WhereAmI?"
                  n203 = local read "WhereAmI?FromBase"() -> (w604:T8)
                  n204 = Get Date/Time In Seconds "GetMiissionCurrentTime"() -> (seconds since 1Jan1904=w615:timestamp)
                  n205 = call "WhereForebrainPerception.vi"("Where? Midbrain"=w604) -> ("(xr,yr)"=w612:cluster{"X":dbl, "Y":dbl}, "Direction"=w598:dbl)  [unwired: 3 in, 2 out]
                  "Robot Position" <- w612
                  n206 = local read "RunAutoMode"() -> (w609:bool)
                  n207 = Greater Or Equal?(x=w598, y=181.0) -> (x >= y?=w602:bool)
                  n208 = To Double Precision Float(number=w615) -> (double precision float=w616:dbl)
                  n209 = Subtract(x=w616, y=w614) -> (x-y=w617:dbl)
                  n210 = Not(x=w610) -> (.not. x?=w619:bool)
                  n211 = call "DrawRobot.vi"("(xr,yr) old"=w613, "(xr,yr) new"=w612, "2D Picture"=w605) -> ("new picture"=→"AutoMissionMap":picture)
                  n212 = local read "SteerAngle"() -> (w607:dbl)
                  n213 = Divide(x=w617, y=60.0) -> (x/y=w611:dbl)
                  "MissionTimeAuto" <- w611
                  n214 = Subtract(x=w598, y=360.0) -> (x-y=w600:dbl)
                  n215 = Select(t=w600, s=w602, f=w598) -> (s? t:f=w599:dbl)
                  n216 = shared-variable "My Computer\\RobotBrainExLibrary.lvlib\\MissionTime"(w611) -> ()  [unwired: 1 in, 1 out]
                  n217 = Bundle("Direction"=w599, "SteerAngle"=w607) -> (→"A Heading":cluster{"Direction":dbl, "SteerAngle":dbl})  [unwired: 1 in]
                  n218 = Wait Until Next ms Multiple(millisecond multiple=u32 50 ("milliseconds to wait")) -> ()  [unwired: 1 out]
                  "Where?" <- w610
                }
                n219 = while {
                  shift-right: [w640] -> _
                  shift-left: _ -> [w639]
                  shift-right: [w622] -> _
                  shift-left: 0.0 ("SteerAngle") -> [w635]
                  stop <- w642 stop-if-true
                  # "needs to put out heading in local coordinates"
                  # "Think"
                  n220 = Not(x=w639) -> (.not. x?=w640:bool)
                  n221 = Or(x="Pause", y="E-Stop") -> (x .or. y?=w626:bool)
                  n222 = local read "WhereAmI?FromBase"() -> (w638:T8)
                  n223 = local read "WhatAroundMeMap?"() -> (w637:cluster{"T":dbl, "Range":dbl, "Bearing":dbl}[])
                  n224 = local read "MDF"() -> (w628:T6)
                  n225 = call "GotoWaypoint.vi"("InhibitIn"=w626, "CurrentSteerAngle"=w635, "WhatAroundMe? Clean"=w637, "WhereAmI? Clean"=w638, "MDF In"=w628) -> ("BehCom"=→"Current Behavior":T9, "MDF Out"=w630:T6, "ActCommand"=→"WayPointAct":dbl[], "Vel"=w623:dbl, "SteerAngle"=w622:dbl)  [unwired: 1 in, 1 out]
                  "SteerAngle" <- w622
                  "A Speed" <- w623
                  n226 = To Long Integer(number=w623) -> (32bit integer=w624:i32)
                  n227 = To Long Integer(number=w622) -> (32bit integer=w621:i32)
                  n228 = local write "MDF"(w630) -> ()
                  n229 = local write "Desired \nVelocity"(w624) -> ()
                  n230 = local read "RunAutoMode"() -> (w642:bool)
                  n231 = local write "Local\nHeading"(w621) -> ()
                  n232 = local read "MDF_Original"() -> (w633:T6)
                  n233 = local read "MDF"() -> (w632:T6)
                  n234 = Select(t=w633, s="Rerun MDF", f=w632) -> (s? t:f=w629:T6)
                  n235 = local write "MDF"(w629) -> ()
                  n236 = Wait Until Next ms Multiple(millisecond multiple=u32 50 ("milliseconds to wait")) -> ()  [unwired: 1 out]
                  "Neo-C" <- w639
                }
                n237 = while {
                  shift-right: [w591] -> _
                  shift-left: _ -> [w593]
                  stop <- w590 stop-if-true
                  # "WhatIsAroundMe?"
                  n238 = local read "WhatAroundMeMap?"() -> (w587:cluster{"T":dbl, "Range":dbl, "Bearing":dbl}[])
                  n239 = call "ProcessLidarData.vi"("WhatAroundMe?MM"=w587) -> ("Collision"=w588:bool, "data array [mag, phase (deg)]"=w592:cluster{"magnitude":dbl, "phase":dbl}[])
                  "CollisionLight 2" <- w588
                  n240 = local read "RunAutoMode"() -> (w590:bool)
                  n241 = call "SimLIDARPlot.vi"("data array [mag, phase (deg)]"=w592) -> ("SONAR"=→"AutoModeLIDAR":picture)  [unwired: 1 in]
                  n242 = Not(x=w593) -> (.not. x?=w591:bool)
                  "What?" <- w591
                  n243 = case shown="True" w588 {
                    frame False {
                      # "No \nBeep"
                    }
                    frame True {
                      n244 = call <vilib>:"Beep.vi"("use system alert? (T)"=TRUE, "duration (msec)"=u32 1000, "frequency (Hz)"=u32 900) -> ()  [unwired: 9 in]
                    }
                  }
                  n245 = Wait Until Next ms Multiple(millisecond multiple=u32 50 ("milliseconds to wait")) -> ()  [unwired: 1 out]
                }
                n246 = while {
                  shift-right: [w585] -> _
                  shift-left: _ -> [w584]
                  stop <- w583 stop-if-true
                  # "HowAmI?"
                  n247 = local read "Battery\nVolts"() -> (w581:i16)
                  n248 = local read "RunAutoMode"() -> (w583:bool)
                  n249 = Not(x=w584) -> (.not. x?=w585:bool)
                  n250 = Divide(x=w581, y=i16 1000) -> (x/y=→"AutoBattery":dbl)
                  n251 = Wait Until Next ms Multiple(millisecond multiple=u32 80 ("milliseconds to wait")) -> ()  [unwired: 1 out]
                  "How?" <- w584
                }
                n252 = while {
                  shift-right: [w578] -> _
                  shift-left: _ -> [w577]
                  stop <- w576 stop-if-true
                  # "calculate desired heading.vi"
                  # "see calc desired\nheading"
                  # "convert to \noutputtin\nDesired v and\nlocal heading"
                  # "chnage arbiter to be -180 to 180"
                  # "Note:\nadd other beh to\narbiter"
                  # "ForebrainAct"
                  n253 = local read "WayPointAct"() -> (w575:dbl[])
                  n254 = local read "RunAutoMode"() -> (w576:bool)
                  n255 = Not(x=w577) -> (.not. x?=w578:bool)
                  n256 = call "ForebrainArbiter.vi"("WaypointInput"=w575) -> ("ForebrainActCom"=w574:dbl[])  [unwired: 14 in]
                  n257 = shared-variable "My Computer\\RobotBrainExLibrary.lvlib\\ActCommand"(w574) -> ()  [unwired: 1 in, 1 out]
                  n258 = Wait Until Next ms Multiple(millisecond multiple=u32 50 ("milliseconds to wait")) -> ()  [unwired: 1 out]
                  "Act" <- w577
                }
              }
              frame #2 {
                w650 = T10."Startup&Shutdown" ("Tab")
                # "Set robot Vel to 0"
                # "Reset latched run\nswitch"
                # "Force control to\nShutdown Case"
                n259 = shared-variable "My Computer\\RobotBrainExLibrary.lvlib\\ForebrainCom"(T11 {"VelCom"=0.0, "BehCom"=enum."OpenFieldTransit"} ("ForebrainCom")) -> ()  [unwired: 1 in, 1 out]
                n260 = local write "RunAutoMode"(TRUE ("RunAutoMode")) -> ()
                n261 = Initialize Array(0.0 ("element"), 90 ("dimension size")) -> (w646:dbl[])
                n262 = shared-variable "My Computer\\RobotBrainExLibrary.lvlib\\ActCommand"(w646) -> ()  [unwired: 1 in, 1 out]
                n263 = shared-variable "My Computer\\RobotBrainExLibrary.lvlib\\Xstart"(200.0 ("Xstart")) -> ()  [unwired: 1 in, 1 out]
                n264 = shared-variable "My Computer\\RobotBrainExLibrary.lvlib\\Ystart"(400.0 ("Ystart")) -> ()  [unwired: 1 in, 1 out]
                n265 = local write "Tab"(w650) -> ()
              }
            }
          }
          frame "Documentation" {
            # "Add:\n1) Blinking lights in each loop to show that they are running"
            # "This mode is just a static data flow picture of the ForeBrain"
            n266 = Wait (ms)(milliseconds to wait=u32 500) -> ()  [unwired: 1 out]
          }
          frame "DebugTHINK" {
            w662 = T10."Startup&Shutdown" ("Tab")
            # "Add:\n1) a button for each midbrain behavior to help in debugging\n2) graph of \"neural\" arbiter brain waves for each actuator\n3) a button for each forebrain behavior"
            # "Put code here in place of delay"
            # "Sends Tab Control\nback to Startup\ncase"
            n267 = Wait (ms)(milliseconds to wait=u32 5000) -> ()  [unwired: 1 out]
            n268 = local write "Tab"(w662) -> ()
          }
          frame "Basic AutoMode" {
            # "last heading"
            # "if we are under a cloud"
            # "Where am I?\nDraw robots current\n location on map"
            n269 = local read "Tug X"() -> (w711:i32)
            n270 = local read "Tug Y"() -> (w712:i32)
            n271 = local read "Current Waypoint"() -> (w684:dbl)
            n272 = Bundle("Tug X"=w711, "Tug Y"=w712) -> (w669:cluster{"Tug X":i32, "Tug Y":i32})  [unwired: 1 in]
            n273 = local read "Buoy Array"() -> (w679:i32[][])
            n274 = case shown="1" "WAYPOINT\n MODE" {
              tunnel: [w719 w730] -> w698
              tunnel: [w720 w728] -> w697
              tunnel: "Destinations Array" -> [w718 w724]
              tunnel: w684 -> [w721 w723]
              tunnel: [w715 w722] -> w664
              frame 1 {
                n275 = Array Size(array=w718) -> (size(s)=w717:i32[])
                n276 = call "MidpointGenerator.vi"("Waypoint"=w721, "Array"=w718) -> ("Y"=w719:dbl, "X"=w720:dbl)
                n277 = Index Array(array=w717, index=0) -> (element=w715:i32)
              }
              frame 0, Default {
                # "Index of Destination Point"
                n278 = Array Size(array=w724) -> (size(s)=w726:i32[])
                n279 = Index Array(array=w724, index (row)=w723, index (col)=1 ("disabled index (col)")) -> (element=w729:i64)
                n280 = Index Array(array=w724, index (row)=w723, index (col)=0 ("index (row)")) -> (element=w731:i64)
                n281 = Index Array(array=w726, index=0) -> (element=w722:i32)
                n282 = To Double Precision Float(number=w729) -> (double precision float=w730:dbl)
                n283 = To Double Precision Float(number=w731) -> (double precision float=w728:dbl)
              }
            }
            "Number Waypoints" <- w664
            n284 = call "DrawRobot.vi"("(xr,yr) old"=w669, "(xr,yr) new"=w669, "2D Picture"=w710) -> ("new picture"=w670:picture)
            n285 = local read "Direction"() -> (w671:dbl)
            n286 = call "BuoyRectifier.vi"("Buoy Array"=w679) -> ("Normalized Buoy Array"=w678:i32[][])
            "Normalized Buoy Array" <- w678
            n287 = call "DrawHeading.vi"("(xr,yr) old"=w669, "Heading"=w671, "2D Picture"=w670) -> ("new picture"=w668:picture)
            n288 = call "DrawWaypoints.vi"("Array"="Destinations Array", "2D Picture"=w668) -> ("new picture"=w682:picture)  [unwired: 1 in]
            n289 = local read "Buoy Array"() -> (w681:i32[][])
            n290 = local write "Buoy Array"(w678) -> ()
            n291 = local read "WhereAmI?FromBase"() -> (w714:T8)
            n292 = call "DrawBuoy.vi"("Array"=w681, "2D Picture"=w682) -> ("new picture"=→"BAM Mission Map":picture)  [unwired: 1 in]
            n293 = call "unpackGates.vi"("Current Waypoint"=w684, "Destinations Array"="Destinations Array") -> ("Past Gate"=w685:i64[], "Current Gate"=w686:i64[])
            n294 = Unbundle(w714) -> ("X"=w675:dbl, "Y"=w687:dbl, "Direction"=w713:dbl)  [unwired: 1 out]
            "Pixel X" <- w675
            "Pixel Y" <- w687
            "Direction" <- w713
            n295 = call "crossedLineWayPoint.vi"("X Boat (Pixel)"=w675, "Y Boat (Pixel)"=w687, "Current Gate"=w686, "Past Gate"=w685) -> ()  [unwired: 1 in, 1 out]
            n296 = call "NearWaypointTest.vi"("Yrobot"=w687, "Xrobot"=w675, "Ywaypoint"=w698, "Xwaypoiny"=w697) -> ("AtWaypoint"=w665:bool)  [unwired: 7 in]
            n297 = call "rudderAngle.vi"("BoatHeading"=w713, "YGoal"=w697, "XGoal"=w698, "Yboat"=w675, "Xboat"=w687) -> ("RudderAngle"=w701:i16)  [unwired: 1 in, 2 out]
            n298 = local read "Number Waypoints"() -> (w693:i32)
            n299 = local read "Current Waypoint"() -> (w694:dbl)
            n300 = Select(t="Heading", s="Manual\nOverride", f=w701) -> (s? t:f=w677:i16)
            n301 = local read "under cloud?"() -> (w667:bool)
            n302 = local read "Battery\nVolts"() -> (w708:i16)
            n303 = Select(t=w674, s=w667, f="Heading") -> (s? t:f=w672:i16)
            n304 = Increment(x=w694) -> (x+1=w695:dbl)
            n305 = Greater Or Equal?(x=w694, y=w693) -> (x >= y?=w691:bool)
            n306 = Select(t=i16 7, s=w691, f=i16 8 ("t")) -> (s? t:f=w699:i16)
            n307 = Divide(x=w708, y=1000) -> (x/y=→"Battery Level":dbl)
            n308 = Select(t=w695, s=w665, f=w694) -> (s? t:f=w696:dbl)
            n309 = local write "Current Waypoint"(w696) -> ()
            n310 = Select(t="Velocity", s="Manual\nOverride", f=w699) -> (s? t:f=w676:i16)
            n311 = local write "Local\nHeading"(w677) -> ()
            n312 = local write "Desired \nVelocity"(w676) -> ()
            n313 = Bundle("RudderAngle"=w677, "t"=w676, "under cloud?"=w667, "Heading"=w672) -> (→"Forebrain to Midbrain":T16)  [unwired: 1 in]
            n314 = local read "Tab"() -> (w704:T3)
          }
        }
        n315 = Not(x=w224) -> (.not. x?=w208:bool)
        "Robot Live" <- w208
      }
      n316 = while {
        tunnel: w61 -> [w170]
        tunnel: w58 -> [w169]
        tunnel: [w166] -> w59
        tunnel: [w165] -> w60
        stop <- w164 continue-if-true
        # "will lock up main  process\nwaiting for return string"
        # "communication loop with NXT"
        # "send a string to the NXT and receive a String in return"
        n317 = local read "Send String"() -> (w162:string)
        "NXT String Sent" <- w162
        n318 = Wait Until Next ms Multiple(millisecond multiple=u32 200) -> ()  [unwired: 1 out]
        n319 = call "XB PC Send.vi"("error in (no error)"=w169, "String"=w162, "VISA resource name"=w170) -> ("error out"=w168:errorcluster, "return count"=→"return count":u32, "VISA resource name out"=w167:refnum<visa-resource-name>)
        n320 = call "XB PC Hear.vi"("VISA resource name"=w167, "error in (no error)"=w168) -> ("VISA resource name out"=w165:refnum<visa-resource-name>, "String Received"=w161:string, "error out"=w166:errorcluster)
        "NXT String Received" <- w161
        n321 = local read "RunRobot"() -> (w164:bool)
        n322 = local write "String Received"(w161) -> ()
      }
      n323 = while {
        tunnel: w57 -> [w189]
        tunnel: w56 -> [w188]
        tunnel: [w187] -> w54
        tunnel: [w186] -> w55
        shift-right: [w180] -> _
        shift-left: _ -> [w179]
        shift-right: [w178] -> _
        shift-left: _ -> [w177]
        shift-left: _ -> [w176]
        shift-left: _ -> [w175]
        shift-left: _ -> [w172]
        shift-left: _ -> [w171]
        stop <- w190 continue-if-true
        w192 = 250  # timeout
        # "Finds and displays tugs position"
        # "runs continuously till program stops"
        # "Comminications with Base Station"
        # "receive string"
        # "If time out, post timeout and\nremove the timeout error"
        # "Read data from the port."
        n324 = Compound Arithmetic op=OR(w177, w176, w175, w171, w172) -> (w174:bool)
        n325 = Wait Until Next ms Multiple(millisecond multiple=u32 1) -> ()  [unwired: 1 out]
        n326 = Not(x=w174) -> (.not. x?=→"under cloud?":bool)
        n327 = UDP Read(connection ID=w189, timeout ms (25000)=w192, 8:w188) -> (data out=w181:string, error out=w193:errorcluster, 3:w186:refnum<k16>)  [unwired: 1 in, 2 out]
        "Base Station String" <- w181
        n328 = local write "Base Station data rec'd"(w181) -> ()
        n329 = Unbundle By Name(w193) -> ("code"=w196:i32)
        n330 = Equal?(x=w196, y=56) -> (x = y?=w194:bool)
        "BS Time Out?" <- w194
        n331 = case shown="True" w194 {
          tunnel: [w203 errorcluster {"status"=FALSE, "code"=0, "source"=""} ("error out")] -> w187
          tunnel: w193 -> [w203 _]
          frame False {
          }
          frame True {
          }
        }
        n332 = call "PC parse the data.vi"("Nav String"=w181, "Tug"="Tug letter") -> ("Buoy locations"=w185:cluster{"regular expression":string, i32, i32}[], "Tug Location"=w183:T17, "Valid?"=w184:bool)  [unwired: 1 out]
        "Valid ?" <- w184
        n333 = local write "Buoy locations"(w185) -> ()
        n334 = case shown="True" w184 {
          tunnel: w183 -> [_ w202]
          frame False {
            # "No \nchange"
          }
          frame True {
            # "New values from BaseStation"
            n335 = shared-variable "My Computer\\RobotBrainExLibrary.lvlib\\MissionTime"() -> (w201:dbl)  [unwired: 1 in, 1 out]
            n336 = Unbundle(w202) -> (w200:i32, w199:i32, w198:i32)  [unwired: 1 out]
            n337 = local write "Tug X"(w200) -> ()
            n338 = local write "Tug Y"(w199) -> ()
            n339 = local write "Tug H"(w198) -> ()
            n340 = Bundle(w201, w200, w199, w198) -> (w197:cluster{dbl, i32, i32, i32})  [unwired: 1 in]
            n341 = local write "WhereAmI?FromBase"(w197) -> ()
          }
        }
        n342 = local read "RunRobot"() -> (w190:bool)
        n343 = Not(x=w179) -> (.not. x?=w180:bool)
        n344 = local read "Valid ?"() -> (w178:bool)
        "udp rate" <- w179
      }
      n345 = while {
        tunnel: w58 -> [_]
        stop <- w116 continue-if-true
        n346 = local read "Upper Midbrain Active"() -> (w115:bool)
        n347 = case shown="True" w115 {
          frame False {
            # "loop timimng \ncontrolled externally"
            # "Send commands to NXT"
            n348 = local read "Desired \nVelocity"() -> (w127:i16)
            n349 = local read "Local\nHeading"() -> (w126:i16)
            n350 = local read "Mode"() -> (w125:i16)
            n351 = case shown="2" w125 {
              tunnel: w127 -> [w130 w141 w148]
              tunnel: w126 -> [w129 w140 w149]
              tunnel: [w131 w136 w144] -> w119
              tunnel: i16 7 ("element") -> [w128 w137 w145]
              frame 0, Default {
                w132 = i16 0 ("element")
                n352 = Build Array(u8 91 ("element"), w128, w129, w130, i16 1 ("element"), w132, w132, w132, w132, w132, u8 93 ("element")) -> (w131:i16[])
              }
              frame 1 {
                w138 = i16 0 ("element")
                n353 = Build Array(u8 91 ("element"), w137, w140, w141, w138, i16 1 ("element"), w138, w138, w138, w138, u8 93 ("element")) -> (w136:i16[])
              }
              frame 2 {
                w146 = i16 0 ("element")
                n354 = Build Array(u8 91 ("element"), w145, w149, w148, w146, w146, i16 1 ("element"), w146, w146, w146, u8 93 ("element")) -> (w144:i16[])
              }
            }
            n355 = Select(t=u8[] [91, 7, 7, 7, 1, 0, 0, 0, 0, 0, 92], s="Soft E-Stop", f=w119) -> (s? t:f=w120:i16[])
            n356 = Add(x=w120, y=u8[] [0, 65, 65, 65, 65, 65, 65, 65, 65, 65, 0]) -> (x+y=w121:i16[])
            n357 = Byte Array To String(unsigned byte array=w121) -> (string=w118:string)
            n358 = local write "Send String"(w118) -> ()
          }
          frame True {
            n359 = local read "WhatAroundMeMap? Filtered"() -> (w155:cluster{"T":dbl, "Range":dbl, "Bearing":dbl}[])
            n360 = local read "Ir distance"() -> (w156:i16)
            n361 = local read "Forebrain to Midbrain"() -> (w153:T1)
            n362 = local read "Direction"() -> (w152:dbl)
            n363 = call "UpperMidbrain.vi"("Boat Heading"=w152, "tweak"="Upper Midbrain Tweaks", "WhatAroundMeMap?"=w155, "SOFT E-STOP"="SOFT E-STOP", "behavior weights"="Midbrain Behavior weights", "ir distance"=w156, "ForeBrain to Midbrain"=w153) -> ("string"=w154:string)  [unwired: 4 in]
            n364 = local write "Send String"(w154) -> ()
          }
        }
        n365 = local read "RunRobot"() -> (w116:bool)
      }
      n366 = while {
        tunnel: w58 -> [_]
        stop <- w86 continue-if-true
        # "Receive information from NXT"
        n367 = local read "String Received"() -> (w91:string)
        n368 = Wait Until Next ms Multiple(millisecond multiple=u32 100) -> ()  [unwired: 1 out]
        n369 = String Subset(string=w91, offset (0)=1, length (rest)=1 ("length (rest)")) -> (substring=w90:string)
        n370 = case shown="Default" w90 {
          tunnel: w91 -> [w92 w100]
          frame Default {
            n371 = Search/Split String(string=w92, search string/char (-)=",", offset (0)=1) -> (substring before match=w94:string)  [unwired: 2 out]
            n372 = Decimal String To Number(string=w94, offset=1) -> (number=w96:i32)  [unwired: 1 in, 1 out]
            n373 = To Word Integer(number=w96) -> (16bit integer=→"Ir distance":i16)
          }
          frame "N" {
            # "0-15"
            # "Parse command \"N\""
            n374 = String Subset(string=w100, offset (0)=2, length (rest)=4 ("length (rest)")) -> (substring=w111:string)
            n375 = String Subset(string=w100, offset (0)=6, length (rest)=3 ("length (rest)")) -> (substring=w107:string)
            n376 = String Subset(string=w100, offset (0)=9, length (rest)=2 ("length (rest)")) -> (substring=w103:string)
            n377 = Decimal String To Number(string=w111) -> (number=w114:i32)  [unwired: 2 in, 1 out]
            n378 = Decimal String To Number(string=w107) -> (number=w106:i32)  [unwired: 2 in, 1 out]
            n379 = Decimal String To Number(string=w103) -> (number=w104:i32)  [unwired: 2 in, 1 out]
            n380 = To Word Integer(number=w114) -> (16bit integer=w110:i16)
            n381 = To Word Integer(number=w106) -> (16bit integer=w105:i16)
            n382 = To Long Integer(number=w104) -> (32bit integer=w99:i32)
            n383 = local write "LidarDist"(w105) -> ()
            n384 = local write "Battery\nVolts"(w110) -> ()
            n385 = local write "IR Index"(w99) -> ()
          }
        }
        n386 = local read "RunRobot"() -> (w86:bool)
      }
      n387 = while {
        shift-right: [w71] -> _
        shift-left: _ -> [w78]
        shift-left: _ -> [w79]
        shift-left: _ -> [w80]
        stop <- w85 continue-if-true
        # "Run Simulated MapDAR"
        n388 = local read "Tug X"() -> (w83:i32)
        n389 = local read "Tug Y"() -> (w82:i32)
        n390 = local read "Tug H"() -> (w81:i32)
        n391 = local read "Buoy Array"() -> (w76:i32[][])
        n392 = call "FilterLidar.vi"("WhatAroundMeMap? Last 2"=w80, "WhatAroundMeMap? Last 3"=w79, "WhatAroundMeMap? Last"=w78) -> ("WhatAroundMeMap?"=→"WhatAroundMeMap? Filtered":cluster{"T":dbl, "Range":dbl, "Bearing":dbl}[])  [unwired: 8 in]
        n393 = Bundle "Bundle"("Tug X"=w83, "Tug Y"=w82, "Tug H"=w81) -> (w84:cluster{"Tug X":i32, "Tug Y":i32, "Tug H":i32})  [unwired: 1 in]
        n394 = call "HindbrainLIDAR_Sim.vi"("Buoys"=w76, "SubPosition"=w84) -> ("WhatAroundMe"=w73:cluster{"T":dbl, "Range":dbl, "Bearing":dbl}[], "WhatAroundMe?Walls"=w72:cluster{"T":dbl, "Range":dbl, "Bearing":dbl}[])
        n395 = Not(x="MapDarWithBuoys?") -> (.not. x?=w74:bool)
        n396 = local read "RunRobot"() -> (w85:bool)
        n397 = Select(t=w72, s=w74, f=w73) -> (s? t:f=w71:cluster{"T":dbl, "Range":dbl, "Bearing":dbl}[])
        "WhatAroundMeMap?" <- w71
      }
    }
    frame #2 {
      # "Close XBee Radio"
      # "Close UDP port"
      # "Realease LIDAR\nMemory"
      # "Reset Run \nSwitch"
      # "Shutdown Robot"
      n398 = call "Pixel_LIDAR_Close.vi"("error in (no error) 2"=w737, "Image"=w738) -> ()  [unwired: 1 in]
      n399 = local write "RunRobot"(TRUE ("RunRobot")) -> ()
      n400 = call "XB PC Close.vi"("error in (no error)"=w735, "VISA resource name"=w736) -> ()
      n401 = UDP Close(connection ID=w734, 8:w733) -> ()  [unwired: 2 out]
      "error out" <- w735
    }
  }
